vi "calculation vi_MD.vi"() -> ()   [LabVIEW 2012]
uses:
  Custom Controls/scan mode main settings tab.ctl
  Custom Controls/display palette control.ctl
  Custom Controls/pixel resolution enum.ctl
  Custom Controls/speed mode type def.ctl
  <vilib>/Utility/miscctls.llb/LVMinMaxIncTypeDef.ctl
  <vilib>/Utility/miscctls.llb/LVOutOfRangeActionTypeDef.ctl
  Custom Controls/experiment type.ctl
  Custom Controls/advanced settings inner tab CTL.ctl
  Custom Controls/MAIN Image panel tab Control type def.ctl
  Custom Controls/Histogram tab.ctl
  GFG/GFGnumericGet.vi
  GFG/GFGfpRefGet.vi
  GFG/GFGbooleanGet.vi
  GFG/GFGDisplayRefsGet.vi
  GFG/GFGImageRefsGet.vi
  GFG/GFG library.lvlib
panel:
  out "error out 3":errorcluster
  in  "String":string
  out "ready for flystart?":bool
  out "error out 2":errorcluster
  out "error out":errorcluster
  out "Source VI":string
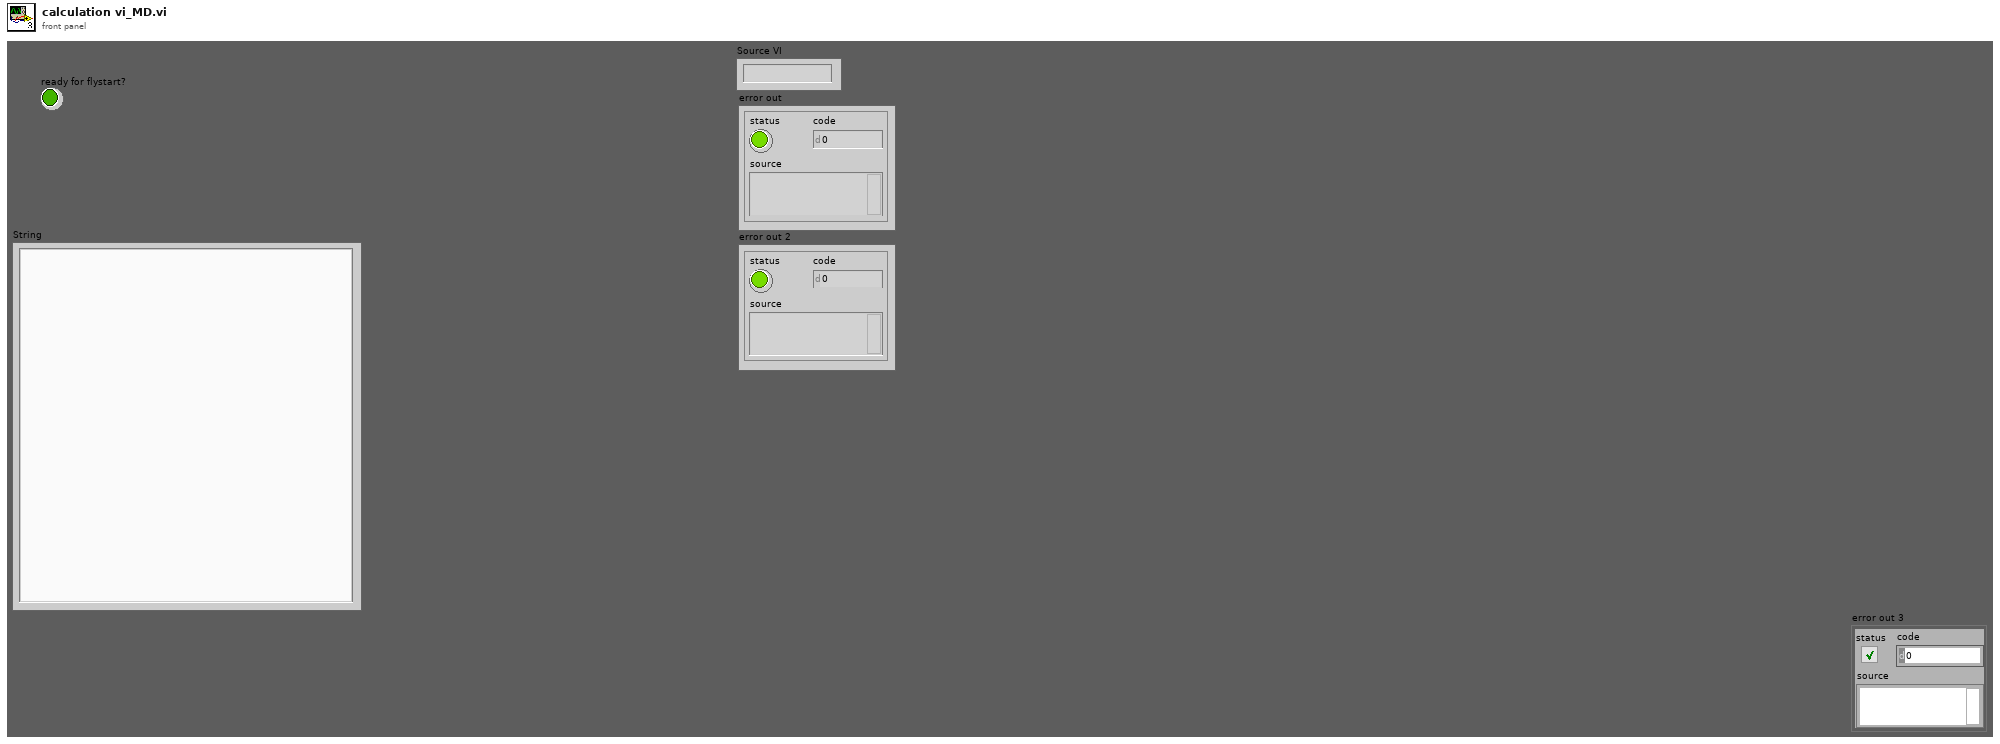
[diagram p1: front panel]
types:
  T1 = typedef "scan mode main settings tab.ctl" = enum32{"2D frame", "2D line scan", "general settings", "Z Stack", "piezo"}
  T2 = typedef "display palette control.ctl" = enum16{"standard", "high clipping red", "low clipping blue", "high and low clipping"}
  T3 = typedef "pixel resolution enum.ctl" = enum16{"   128 x 128", "   256 x 128", "   256 x 256", "   512 x  64", "   512 x 128", "   512 x 256", "   512 x 512", "  1024 x 512", "  1024 x 1024", "   arbitrary"}
  T4 = enum8{"Enabled", "Disabled", "Disabled and Grayed Out"}
  T5 = typedef "LVOutOfRangeActionTypeDef.ctl" = cluster{"Out of Range Action Minimum":u8, "Out of Range Action Maximum":u8, "Out of Range Action Increment":u8}
  T6 = typedef "LVMinMaxIncTypeDef.ctl" = cluster{"Minimum":dbl, "Maximum":dbl, "Increment":dbl}
  T7 = cluster{"xyvoltagefor2frames":dbl[][][], "x.pixels":dbl, "nomin.x.pixels":dbl, "y.pixels":dbl, "fill.fraction":dbl, "x.bidirectional":bool, "y.bidirectional":bool}
  T8 = typedef "experiment type.ctl" = string
  T9 = enum32{"Page Enabled", "Page Disabled", "Page Disabled & Grayed"}
  T10 = typedef "advanced settings inner tab CTL.ctl" = enum32{"arb. frames", "AO", "AI", "channels", "trigger", "Zstack data"}
  T11 = typedef "MAIN Image panel tab Control type def.ctl" = enum32{"Channel 1", "Channel 2", "Channel 3", "Channel 4", "all channels", "RGB overlay", "ROI", "arbitrary line scan"}
  T12 = typedef "Histogram tab.ctl" = enum32{"hist Ch 1", "hist Ch 4", "hist Ch 3", "hist Ch 2"}
  T13 = cluster{"WaveformChartRef":refnum<vi>, "DigitalRef":refnum<vi>, "ArrayRef":refnum<vi>, "TabControlRef":refnum<vi>, "EnumRef":refnum<vi>, "RingRef":refnum<vi>, "BooleanRef":refnum<vi>, "KnobRef":refnum<vi>, "SlideRef":refnum<vi>, "PathRef":refnum<vi>, "StringRef":refnum<vi>, "ComboBox":refnum<vi>, "WaveformGraphRef":refnum<vi>}
  T14 = cluster{"Channel 1 small":refnum<vi>, "Channel 2 small":refnum<vi>, "Channel 3 small":refnum<vi>, "Channel 4 small":refnum<vi>, "Channel 1 large":refnum<vi>, "Channel 2 large":refnum<vi>, "Channel 3 large":refnum<vi>, "Channel 4 large":refnum<vi>, "RGB overlay":refnum<vi>, "ROI Image display":refnum<vi>, "arb line scan display":refnum<vi>, "Channel 5 large":refnum<vi>}
  T15 = typedef "IMAQ Image.ctl" = refnum<image>
  T16 = cluster{"Channel 1 small":T15, "Channel 2 small":T15, "Channel 3 small":T15, "Channel 4 small":T15, "Channel 1 large":T15, "Channel 2 large":T15, "Channel 3 large":T15, "Channel 4 large":T15, "RGB overlay":T15, "ROI Image display":T15, "arb line scan display":T15, "Channel 5 large":T15}
  T17 = typedef "speed mode type def.ctl" = u16
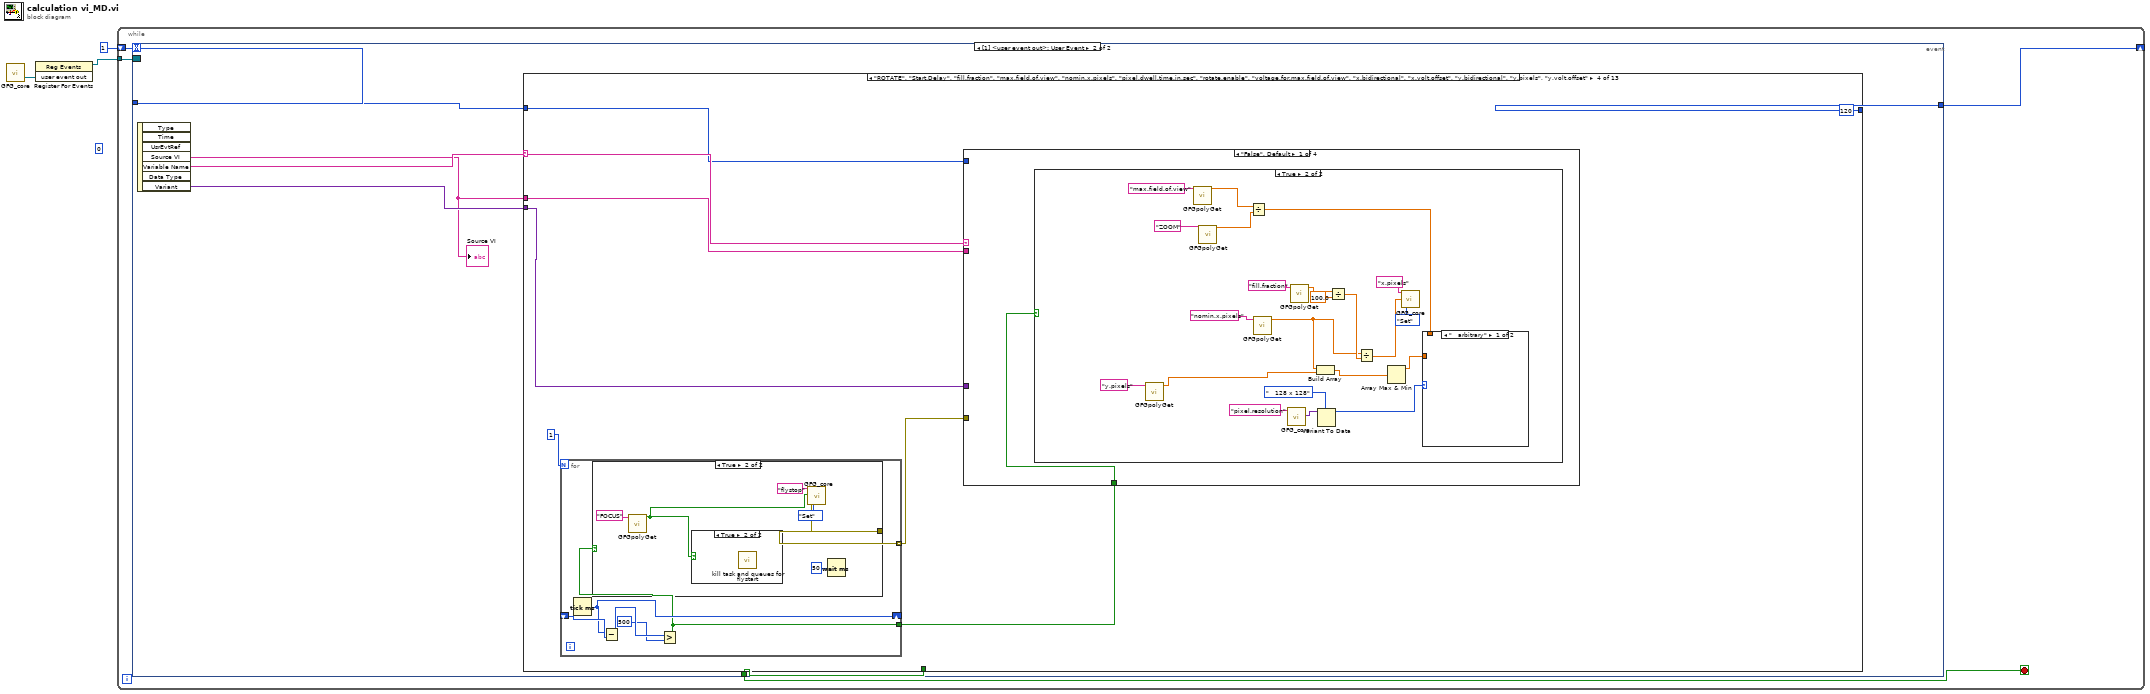
[diagram p0: block diagram]
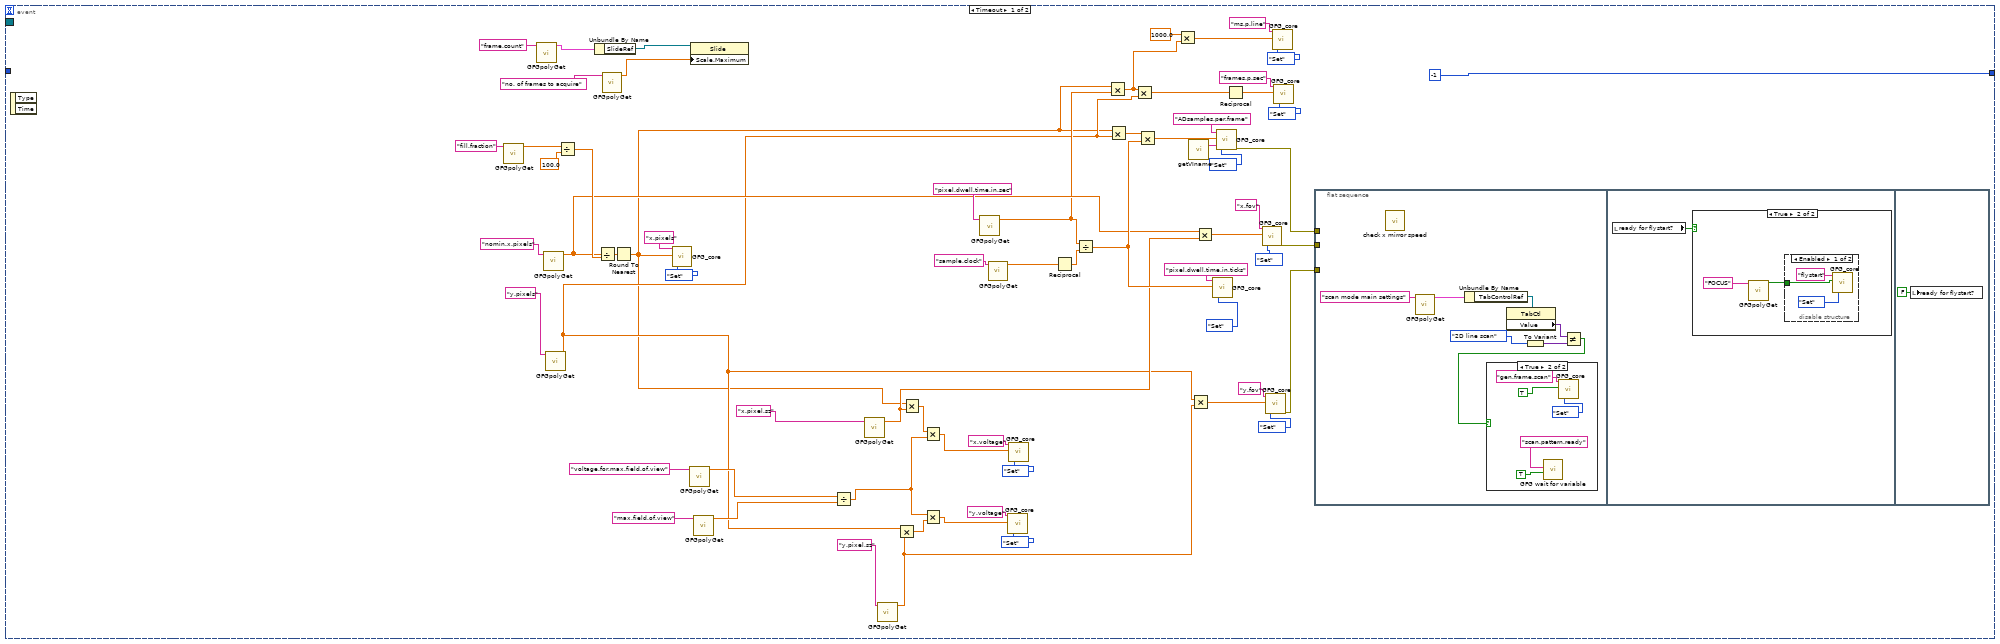
[diagram p2: hidden frame]
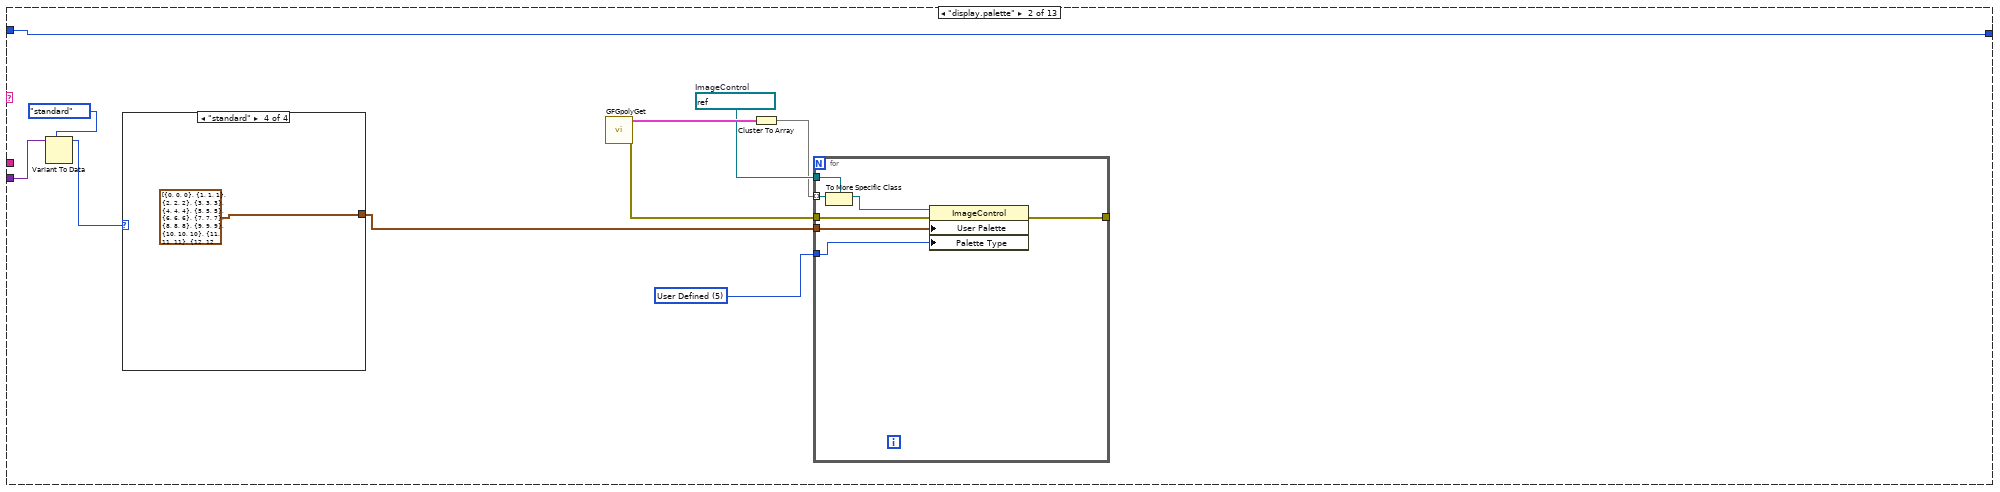
[diagram p7: hidden frame]
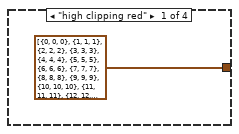
[diagram p8: hidden frame]
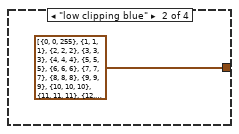
[diagram p9: hidden frame]
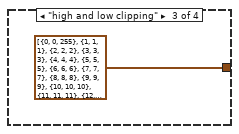
[diagram p10: hidden frame]
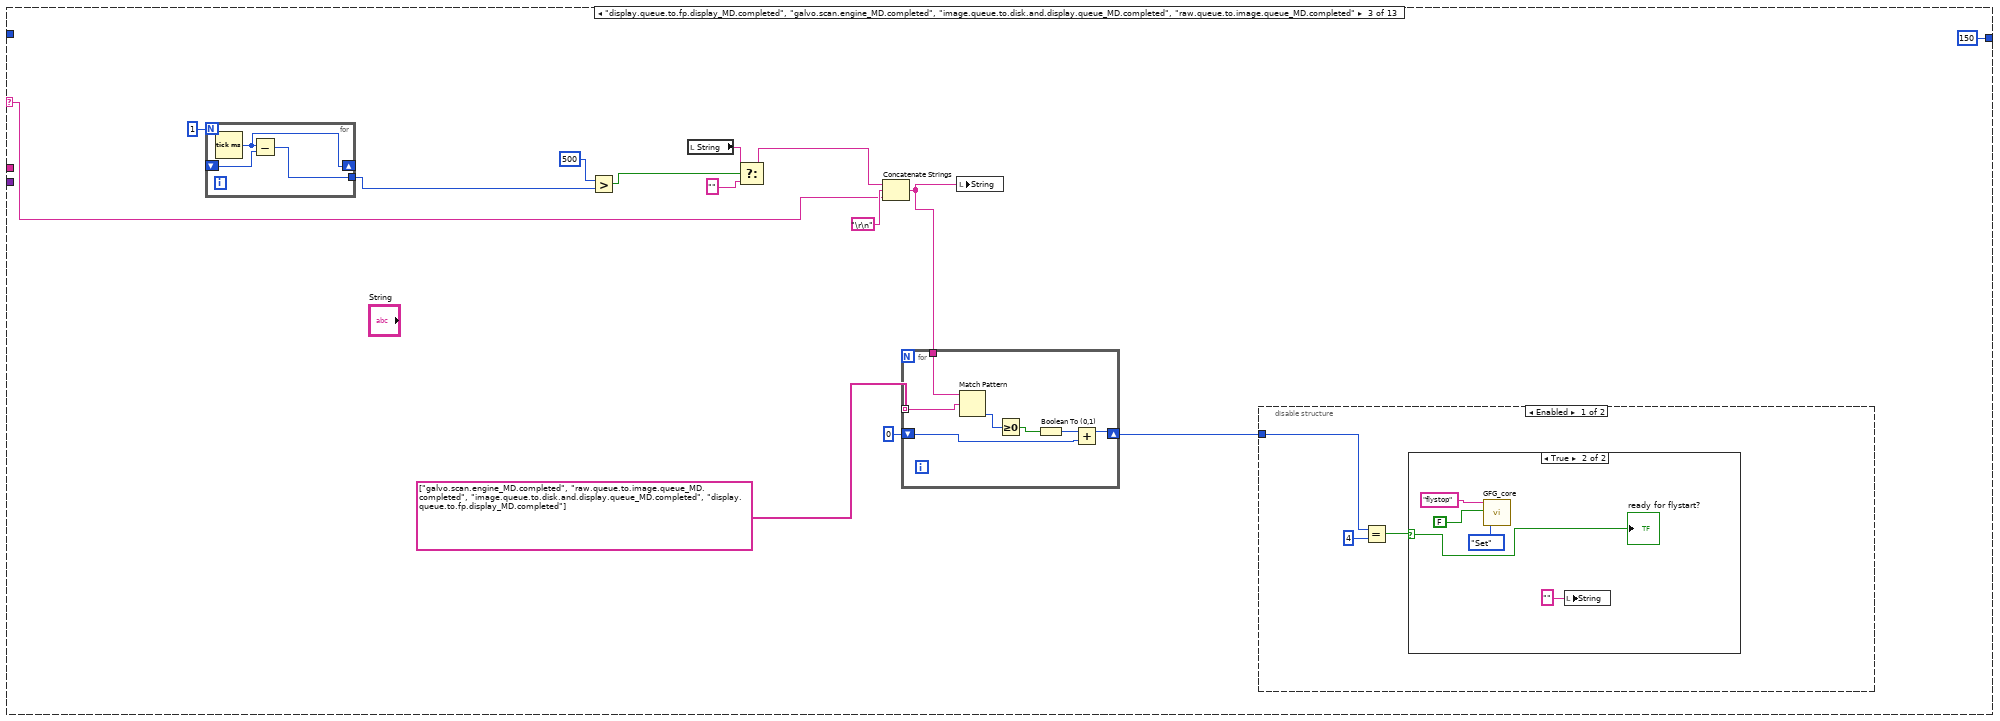
[diagram p11: hidden frame]
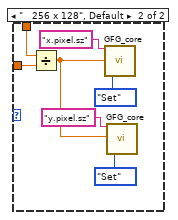
[diagram p17: hidden frame]
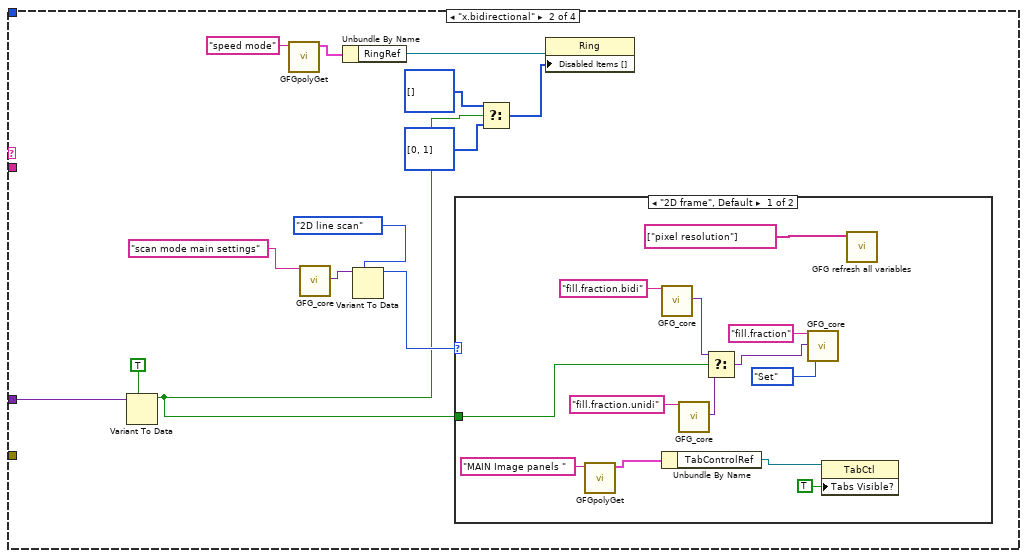
[diagram p18: hidden frame]
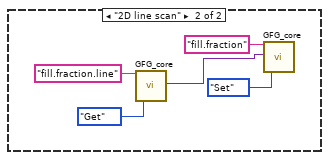
[diagram p19: hidden frame]
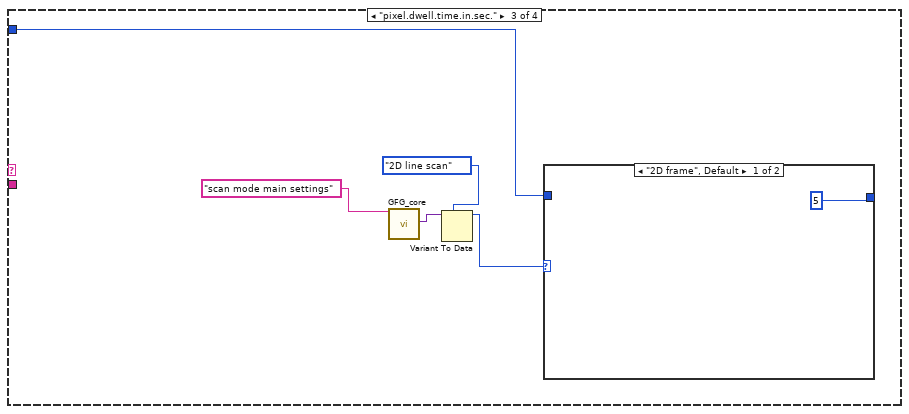
[diagram p20: hidden frame]
diagram:
  (unwired) 0
  n1 = call "GFG_core.vi"() -> ("user event out"=w3:refnum<user-event>)  [unwired: 13 in, 6 out]
  n2 = register-events(w3) -> (reference out=w2:refnum<event-registration>)  [unwired: 2 in, 1 out]
  n3 = while {
    tunnel: w2 -> [w7]
    shift-right: [w5] -> _
    shift-left: 1 -> [w4]
    stop <- w6 stop-if-true
    n4 = event shown="[1] <user event out>: User Event" {
      selector: w7 -> [_ _]
      dyn-events: _ -> [_ _]
      timeout: w4 -> [_ _]
      tunnel: [_ w97] -> w6
      tunnel: [-1 w95] -> w5
      tunnel: w4 -> [_ w94]
      event Timeout {
        n5 = event-data() -> ()  [unwired: 1 in, 2 out]
        n6 = call-poly "GFGpolyGet.vi"("Variable Name in"="fill.fraction") -> ("Numeric"=w53:dbl)  [unwired: 9 in, 1 out]
        n7 = call-poly "GFGpolyGet.vi"("Variable Name in"="frame.count") -> ("output cluster"=w14:T13)  [unwired: 9 in, 1 out]
        n8 = call-poly "GFGpolyGet.vi"("Variable Name in"="nomin.x.pixels") -> ("Numeric"=w29:dbl)  [unwired: 9 in, 1 out]
        n9 = call-poly "GFGpolyGet.vi"("Variable Name in"="y.pixels") -> ("Numeric"=w17:dbl)  [unwired: 9 in, 1 out]
        n10 = Divide(x=w53, y=100.0) -> (x/y=w49:dbl)
        n11 = Unbundle By Name(w14) -> ("SlideRef"=w13:refnum<vi>)
        n12 = Divide(x=w29, y=w49) -> (x/y=w30:dbl)
        n13 = call-poly "GFGpolyGet.vi"("Variable Name in"="no. of frames to acquire") -> ("Numeric"=w11:dbl)  [unwired: 9 in, 1 out]
        n14 = Round To Nearest(number=w30) -> (nearest integer value=w16:dbl)
        n15 = call "GFG_core.vi"("Variable Name in"="x.pixels", "Variant in"=w16, "Action"=enum16{"Init", "Set", "Get"}."Set") -> ()  [unwired: 10 in, 7 out]
        n16 = call-poly "GFGpolyGet.vi"("Variable Name in"="voltage.for.max.field.of.view") -> ("Numeric"=w44:dbl)  [unwired: 9 in, 1 out]
        n17 = property class="Slide"(reference=w13, "Scale.Maximum"=w11) -> ()  [unwired: 1 in, 2 out]
        n18 = call-poly "GFGpolyGet.vi"("Variable Name in"="max.field.of.view") -> ("Numeric"=w45:dbl)  [unwired: 9 in, 1 out]
        n19 = Divide(x=w44, y=w45) -> (x/y=w43:dbl)
        n20 = call-poly "GFGpolyGet.vi"("Variable Name in"="x.pixel.sz") -> ("Numeric"=w35:dbl)  [unwired: 9 in, 1 out]
        n21 = call-poly "GFGpolyGet.vi"("Variable Name in"="y.pixel.sz") -> ("Numeric"=w33:dbl)  [unwired: 9 in, 1 out]
        n22 = Multiply(x=w17, y=w33) -> (x*y=w32:dbl)
        n23 = Multiply(x=w16, y=w35) -> (x*y=w34:dbl)
        n24 = Multiply(x=w34, y=w43) -> (x*y=w38:dbl)
        n25 = Multiply(x=w43, y=w32) -> (x*y=w37:dbl)
        n26 = call-poly "GFGpolyGet.vi"("Variable Name in"="pixel.dwell.time.in.sec") -> ("Numeric"=w21:dbl)  [unwired: 9 in, 1 out]
        n27 = call-poly "GFGpolyGet.vi"("Variable Name in"="sample.clock") -> ("Numeric"=w31:dbl)  [unwired: 9 in, 1 out]
        n28 = call "GFG_core.vi"("Variable Name in"="y.voltage", "Variant in"=w37, "Action"=enum16{"Init", "Set", "Get"}."Set") -> ()  [unwired: 10 in, 7 out]
        n29 = call "GFG_core.vi"("Variable Name in"="x.voltage", "Variant in"=w38, "Action"=enum16{"Init", "Set", "Get"}."Set") -> ()  [unwired: 10 in, 7 out]
        n30 = Reciprocal(x=w31) -> (1/x=w60:dbl)
        n31 = Divide(x=w21, y=w60) -> (x/y=w56:dbl)
        n32 = Multiply(x=w16, y=w21) -> (x*y=w20:dbl)
        n33 = Multiply(x=w16, y=w17) -> (x*y=w28:dbl)
        n34 = Multiply(x=w20, y=w17) -> (x*y=w23:dbl)
        n35 = Multiply(x=w28, y=w56) -> (x*y=w72:dbl)
        n36 = Multiply(x=1000.0, y=w20) -> (x*y=w18:dbl)
        n37 = call "getVIname.vi"() -> ("VI name"=w70:string)  [unwired: 19 in]
        n38 = Multiply(x=w17, y=w33) -> (x*y=w62:dbl)
        n39 = Multiply(x=w29, y=w35) -> (x*y=w65:dbl)
        n40 = call "GFG_core.vi"("Variable Name in"="pixel.dwell.time.in.ticks", "Variant in"=w56, "Action"=enum16{"Init", "Set", "Get"}."Set") -> ()  [unwired: 10 in, 7 out]
        n41 = call "GFG_core.vi"("Variable Name in"="ADsamples.per.frame", "Variant in"=w72, "Source VI"=w70, "Action"=enum16{"Init", "Set", "Get"}."Set") -> ("error out"=w10:errorcluster)  [unwired: 9 in, 6 out]
        n42 = Reciprocal(x=w23) -> (1/x=w22:dbl)
        n43 = call "GFG_core.vi"("Variable Name in"="x.fov", "Variant in"=w65, "Action"=enum16{"Init", "Set", "Get"}."Set") -> ("error out"=w9:errorcluster)  [unwired: 10 in, 6 out]
        n44 = call "GFG_core.vi"("Variable Name in"="y.fov", "Variant in"=w62, "Action"=enum16{"Init", "Set", "Get"}."Set") -> ("error out"=w8:errorcluster)  [unwired: 10 in, 6 out]
        n45 = call "GFG_core.vi"("Variable Name in"="ms.p.line", "Variant in"=w18, "Action"=enum16{"Init", "Set", "Get"}."Set") -> ()  [unwired: 10 in, 7 out]
        n46 = call "GFG_core.vi"("Variable Name in"="frames.p.sec", "Variant in"=w22, "Action"=enum16{"Init", "Set", "Get"}."Set") -> ()  [unwired: 10 in, 7 out]
        n47 = flat-sequence {
          tunnel: w10 -> [_]
          tunnel: w9 -> [_]
          tunnel: w8 -> [_]
          frame #0 {
            n48 = call "check x mirror speed.vi"() -> ()  [unwired: 11 in, 1 out]
            n49 = call-poly "GFGpolyGet.vi"("Variable Name in"="scan mode main settings") -> ("output cluster"=w78:T13)  [unwired: 9 in, 1 out]
            n50 = Unbundle By Name(w78) -> ("TabControlRef"=w80:refnum<vi>)
            n51 = property class="TabCtl"(reference=w80) -> ("Value"=w77:variant)  [unwired: 1 in, 2 out]
            n52 = To Variant(anything=scan_mode_main_settings_tab."2D line scan" ("scan mode main settings")) -> (Variant=w75:variant)
            n53 = Not Equal?(x=w77, y=w75) -> (x != y?=w74:bool)
            n54 = case shown="True" w74 {
              frame False {
              }
              frame True {
                n55 = call "GFG wait for variable.vi"("Variant"=TRUE, "Variable Name"="scan.pattern.ready" ("Variable Name in")) -> ()  [unwired: 10 in]
                n56 = call "GFG_core.vi"("Variable Name in"="gen.frame.scan", "Variant in"=TRUE, "Action"=enum16{"Init", "Set", "Get"}."Set") -> ()  [unwired: 10 in, 7 out]
              }
            }
          }
          frame #1 {
            n57 = local read "ready for flystart?"() -> (w86:bool)
            n58 = case shown="True" w86 {
              frame False {
              }
              frame True {
                n59 = call-poly "GFGpolyGet.vi"("Variable Name in"="FOCUS") -> ("Boolean"=w87:bool)  [unwired: 10 in]
                n60 = disable-structure shown="Enabled" {
                  disable-tunnel: w87 -> [w89 _]
                  frame Enabled {
                    n61 = call "GFG_core.vi"("Variable Name in"="flystart", "Variant in"=w89, "Action"=enum16{"Init", "Set", "Get"}."Set") -> ()  [unwired: 10 in, 7 out]
                  }
                  frame Disabled {
                  }
                }
              }
            }
          }
          frame #2 {
            n62 = local write "ready for flystart?"(FALSE ("ready for flystart?")) -> ()
          }
        }
      }
      event User Event {
        n63 = event-data() -> ("Source VI"=w93:string, "Variable Name"=w98:string, "Variant"=w96:variant)  [unwired: 1 in, 4 out]
        "Source VI" <- w93
        n64 = case shown="\"ROTATE\", \"Start.Delay\", \"fill.fraction\", \"max.field.of.view\", \"nomin.x.pixels\", \"pixel.dwell.time.in.sec\", \"rotate.enable\", \"voltage.for.max.field.of.view\", \"x.bidirectional\", \"x.volt.offset\", \"y.bidirectional\", \"y.pixels\", \"y.volt.offset\"" w98 {
          selector: w98 -> [_ _ w122 w160 _ _ _ w285 _ _ _ _ _]
          tunnel: [_ _ _ _ _ _ _ _ _ _ _ _ TRUE] -> w97
          tunnel: w96 -> [_ w104 _ w159 _ w269 _ w287 _ w418 w478 w512 _]
          tunnel: [w99 w100 150 120 50 w267 w276 120 w404 w414 w475 w513 w514] -> w95
          tunnel: w94 -> [w99 w100 _ w158 _ w267 w276 _ w404 w415 w476 w513 w514]
          tunnel: w93 -> [_ _ _ w157 _ _ _ _ _ _ _ _ _]
          frame "False", Default {
          }
          frame "display.palette" {
            w105 = u32 5 items=["Grayscale", "Binary", "Gradient", "Rainbow", "Temperature", "User Defined"] ("Palette:Palette Type")
            w107 = refnum<vi> refnum  # ImageControl
            n65 = Variant To Data(type=display_palette_control."standard" ("display palette"), Variant=w104) -> (data=w102:T2)  [unwired: 1 in, 1 out]
            n66 = case shown="\"standard\"" w102 {
              tunnel: [cluster{"Red":u8, "Green":u8, "Blue":u8}[] [{"Red"=0, "Green"=0, "Blue"=0}, {"Red"=1, "Green"=1, "Blue"=1}, {"Red"=2, "Green"=2, "Blue"=2}, {"Red"=3, "Green"=3, "Blue"=3}, {"Red"=4, "Green"=4, "Blue"=4}, {"Red"=5, "Green"=5, "Blue"=5}, {"Red"=6, "Green"=6, "Blue"=6}, {"Red"=7, "Green"=7, "Blue"=7}, {"Red"=8, "Green"=8, "Blue"=8}, {"Red"=9, "Green"=9, "Blue"=9}, {"Red"=10, "Green"=10, "Blue"=10}, {"Red"=11, "Green"=11, "Blue"=11}, {"Red"=12, "Green"=12, "Blue"=12}, {"Red"=13, "Green"=13, "Blue"=13}, {"Red"=14, "Green"=14, "Blue"=14}, {"Red"=15, "Green"=15, "Blue"=15}, {"Red"=16, "Green"=16, "Blue"=16}, {"Red"=17, "Green"=17, "Blue"=17}, {"Red"=18, "Green"=18, "Blue"=18}, {"Red"=19, "Green"=19, "Blue"=19}, {"Red"=20, "Green"=20, "Blue"=20}, {"Red"=21, "Green"=21, "Blue"=21}, {"Red"=22, "Green"=22, "Blue"=22}, {"Red"=23, "Green"=23, "Blue"=23}, {"Red"=24, "Green"=24, "Blue"=24}, {"Red"=25, "Green"=25, "Blue"=25}, {"Red"=26, "Green"=26, "Blue"=26}, {"Red"=27, "Green"=27, "Blue"=27}, {"Red"=28, "Green"=28, "Blue"=28}, {"Red"=29, "Green"=29, "Blue"=29}, {"Red"=30, "Green"=30, "Blue"=30}, {"Red"=31, "Green"=31, "Blue"=31}, {"Red"=32, "Green"=32, "Blue"=32}, {"Red"=33, "Green"=33, "Blue"=33}, {"Red"=34, "Green"=34, "Blue"=34}, {"Red"=35, "Green"=35, "Blue"=35}, {"Red"=36, "Green"=36, "Blue"=36}, {"Red"=37, "Green"=37, "Blue"=37}, {"Red"=38, "Green"=38, "Blue"=38}, {"Red"=39, "Green"=39, "Blue"=39}, {"Red"=40, "Green"=40, "Blue"=40}, {"Red"=41, "Green"=41, "Blue"=41}, {"Red"=42, "Green"=42, "Blue"=42}, {"Red"=43, "Green"=43, "Blue"=43}, {"Red"=44, "Green"=44, "Blue"=44}, {"Red"=45, "Green"=45, "Blue"=45}, {"Red"=46, "Green"=46, "Blue"=46}, {"Red"=47, "Green"=47, "Blue"=47}, {"Red"=48, "Green"=48, "Blue"=48}, {"Red"=49, "Green"=49, "Blue"=49}, {"Red"=50, "Green"=50, "Blue"=50}, {"Red"=51, "Green"=51, "Blue"=51}, {"Red"=52, "Green"=52, "Blue"=52}, {"Red"=53, "Green"=53, "Blue"=53}, {"Red"=54, "Green"=54, "Blue"=54}, {"Red"=55, "Green"=55, "Blue"=55}, {"Red"=56, "Green"=56, "Blue"=56}, {"Red"=57, "Green"=57, "Blue"=57}, {"Red"=58, "Green"=58, "Blue"=58}, {"Red"=59, "Green"=59, "Blue"=59}, {"Red"=60, "Green"=60, "Blue"=60}, {"Red"=61, "Green"=61, "Blue"=61}, {"Red"=62, "Green"=62, "Blue"=62}, {"Red"=63, "Green"=63, "Blue"=63}, {"Red"=64, "Green"=64, "Blue"=64}, {"Red"=65, "Green"=65, "Blue"=65}, {"Red"=66, "Green"=66, "Blue"=66}, {"Red"=67, "Green"=67, "Blue"=67}, {"Red"=68, "Green"=68, "Blue"=68}, {"Red"=69, "Green"=69, "Blue"=69}, {"Red"=70, "Green"=70, "Blue"=70}, {"Red"=71, "Green"=71, "Blue"=71}, {"Red"=72, "Green"=72, "Blue"=72}, {"Red"=73, "Green"=73, "Blue"=73}, {"Red"=74, "Green"=74, "Blue"=74}, {"Red"=75, "Green"=75, "Blue"=75}, {"Red"=76, "Green"=76, "Blue"=76}, {"Red"=77, "Green"=77, "Blue"=77}, {"Red"=78, "Green"=78, "Blue"=78}, {"Red"=79, "Green"=79, "Blue"=79}, {"Red"=80, "Green"=80, "Blue"=80}, {"Red"=81, "Green"=81, "Blue"=81}, {"Red"=82, "Green"=82, "Blue"=82}, {"Red"=83, "Green"=83, "Blue"=83}, {"Red"=84, "Green"=84, "Blue"=84}, {"Red"=85, "Green"=85, "Blue"=85}, {"Red"=86, "Green"=86, "Blue"=86}, {"Red"=87, "Green"=87, "Blue"=87}, {"Red"=88, "Green"=88, "Blue"=88}, {"Red"=89, "Green"=89, "Blue"=89}, {"Red"=90, "Green"=90, "Blue"=90}, {"Red"=91, "Green"=91, "Blue"=91}, {"Red"=92, "Green"=92, "Blue"=92}, {"Red"=93, "Green"=93, "Blue"=93}, {"Red"=94, "Green"=94, "Blue"=94}, {"Red"=95, "Green"=95, "Blue"=95}, {"Red"=96, "Green"=96, "Blue"=96}, {"Red"=97, "Green"=97, "Blue"=97}, {"Red"=98, "Green"=98, "Blue"=98}, {"Red"=99, "Green"=99, "Blue"=99}, {"Red"=100, "Green"=100, "Blue"=100}, {"Red"=101, "Green"=101, "Blue"=101}, {"Red"=102, "Green"=102, "Blue"=102}, {"Red"=103, "Green"=103, "Blue"=103}, {"Red"=104, "Green"=104, "Blue"=104}, {"Red"=105, "Green"=105, "Blue"=105}, {"Red"=106, "Green"=106, "Blue"=106}, {"Red"=107, "Green"=107, "Blue"=107}, {"Red"=108, "Green"=108, "Blue"=108}, {"Red"=109, "Green"=109, "Blue"=109}, {"Red"=110, "Green"=110, "Blue"=110}, {"Red"=111, "Green"=111, "Blue"=111}, {"Red"=112, "Green"=112, "Blue"=112}, {"Red"=113, "Green"=113, "Blue"=113}, {"Red"=114, "Green"=114, "Blue"=114}, {"Red"=115, "Green"=115, "Blue"=115}, {"Red"=116, "Green"=116, "Blue"=116}, {"Red"=117, "Green"=117, "Blue"=117}, {"Red"=118, "Green"=118, "Blue"=118}, {"Red"=119, "Green"=119, "Blue"=119}, {"Red"=120, "Green"=120, "Blue"=120}, {"Red"=121, "Green"=121, "Blue"=121}, {"Red"=122, "Green"=122, "Blue"=122}, {"Red"=123, "Green"=123, "Blue"=123}, {"Red"=124, "Green"=124, "Blue"=124}, {"Red"=125, "Green"=125, "Blue"=125}, {"Red"=126, "Green"=126, "Blue"=126}, {"Red"=127, "Green"=127, "Blue"=127}, {"Red"=128, "Green"=128, "Blue"=128}, {"Red"=129, "Green"=129, "Blue"=129}, {"Red"=130, "Green"=130, "Blue"=130}, {"Red"=131, "Green"=131, "Blue"=131}, {"Red"=132, "Green"=132, "Blue"=132}, {"Red"=133, "Green"=133, "Blue"=133}, {"Red"=134, "Green"=134, "Blue"=134}, {"Red"=135, "Green"=135, "Blue"=135}, {"Red"=136, "Green"=136, "Blue"=136}, {"Red"=137, "Green"=137, "Blue"=137}, {"Red"=138, "Green"=138, "Blue"=138}, {"Red"=139, "Green"=139, "Blue"=139}, {"Red"=140, "Green"=140, "Blue"=140}, {"Red"=141, "Green"=141, "Blue"=141}, {"Red"=142, "Green"=142, "Blue"=142}, {"Red"=143, "Green"=143, "Blue"=143}, {"Red"=144, "Green"=144, "Blue"=144}, {"Red"=145, "Green"=145, "Blue"=145}, {"Red"=146, "Green"=146, "Blue"=146}, {"Red"=147, "Green"=147, "Blue"=147}, {"Red"=148, "Green"=148, "Blue"=148}, {"Red"=149, "Green"=149, "Blue"=149}, {"Red"=150, "Green"=150, "Blue"=150}, {"Red"=151, "Green"=151, "Blue"=151}, {"Red"=152, "Green"=152, "Blue"=152}, {"Red"=153, "Green"=153, "Blue"=153}, {"Red"=154, "Green"=154, "Blue"=154}, {"Red"=155, "Green"=155, "Blue"=155}, {"Red"=156, "Green"=156, "Blue"=156}, {"Red"=157, "Green"=157, "Blue"=157}, {"Red"=158, "Green"=158, "Blue"=158}, {"Red"=159, "Green"=159, "Blue"=159}, {"Red"=160, "Green"=160, "Blue"=160}, {"Red"=161, "Green"=161, "Blue"=161}, {"Red"=162, "Green"=162, "Blue"=162}, {"Red"=163, "Green"=163, "Blue"=163}, {"Red"=164, "Green"=164, "Blue"=164}, {"Red"=165, "Green"=165, "Blue"=165}, {"Red"=166, "Green"=166, "Blue"=166}, {"Red"=167, "Green"=167, "Blue"=167}, {"Red"=168, "Green"=168, "Blue"=168}, {"Red"=169, "Green"=169, "Blue"=169}, {"Red"=170, "Green"=170, "Blue"=170}, {"Red"=171, "Green"=171, "Blue"=171}, {"Red"=172, "Green"=172, "Blue"=172}, {"Red"=173, "Green"=173, "Blue"=173}, {"Red"=174, "Green"=174, "Blue"=174}, {"Red"=175, "Green"=175, "Blue"=175}, {"Red"=176, "Green"=176, "Blue"=176}, {"Red"=177, "Green"=177, "Blue"=177}, {"Red"=178, "Green"=178, "Blue"=178}, {"Red"=179, "Green"=179, "Blue"=179}, {"Red"=180, "Green"=180, "Blue"=180}, {"Red"=181, "Green"=181, "Blue"=181}, {"Red"=182, "Green"=182, "Blue"=182}, {"Red"=183, "Green"=183, "Blue"=183}, {"Red"=184, "Green"=184, "Blue"=184}, {"Red"=185, "Green"=185, "Blue"=185}, {"Red"=186, "Green"=186, "Blue"=186}, {"Red"=187, "Green"=187, "Blue"=187}, {"Red"=188, "Green"=188, "Blue"=188}, {"Red"=189, "Green"=189, "Blue"=189}, {"Red"=190, "Green"=190, "Blue"=190}, {"Red"=191, "Green"=191, "Blue"=191}, {"Red"=192, "Green"=192, "Blue"=192}, {"Red"=193, "Green"=193, "Blue"=193}, {"Red"=194, "Green"=194, "Blue"=194}, {"Red"=195, "Green"=195, "Blue"=195}, {"Red"=196, "Green"=196, "Blue"=196}, {"Red"=197, "Green"=197, "Blue"=197}, {"Red"=198, "Green"=198, "Blue"=198}, {"Red"=199, "Green"=199, "Blue"=199}, {"Red"=200, "Green"=200, "Blue"=200}, {"Red"=201, "Green"=201, "Blue"=201}, {"Red"=202, "Green"=202, "Blue"=202}, {"Red"=203, "Green"=203, "Blue"=203}, {"Red"=204, "Green"=204, "Blue"=204}, {"Red"=205, "Green"=205, "Blue"=205}, {"Red"=206, "Green"=206, "Blue"=206}, {"Red"=207, "Green"=207, "Blue"=207}, {"Red"=208, "Green"=208, "Blue"=208}, {"Red"=209, "Green"=209, "Blue"=209}, {"Red"=210, "Green"=210, "Blue"=210}, {"Red"=211, "Green"=211, "Blue"=211}, {"Red"=212, "Green"=212, "Blue"=212}, {"Red"=213, "Green"=213, "Blue"=213}, {"Red"=214, "Green"=214, "Blue"=214}, {"Red"=215, "Green"=215, "Blue"=215}, {"Red"=216, "Green"=216, "Blue"=216}, {"Red"=217, "Green"=217, "Blue"=217}, {"Red"=218, "Green"=218, "Blue"=218}, {"Red"=219, "Green"=219, "Blue"=219}, {"Red"=220, "Green"=220, "Blue"=220}, {"Red"=221, "Green"=221, "Blue"=221}, {"Red"=222, "Green"=222, "Blue"=222}, {"Red"=223, "Green"=223, "Blue"=223}, {"Red"=224, "Green"=224, "Blue"=224}, {"Red"=225, "Green"=225, "Blue"=225}, {"Red"=226, "Green"=226, "Blue"=226}, {"Red"=227, "Green"=227, "Blue"=227}, {"Red"=228, "Green"=228, "Blue"=228}, {"Red"=229, "Green"=229, "Blue"=229}, {"Red"=230, "Green"=230, "Blue"=230}, {"Red"=231, "Green"=231, "Blue"=231}, {"Red"=232, "Green"=232, "Blue"=232}, {"Red"=233, "Green"=233, "Blue"=233}, {"Red"=234, "Green"=234, "Blue"=234}, {"Red"=235, "Green"=235, "Blue"=235}, {"Red"=236, "Green"=236, "Blue"=236}, {"Red"=237, "Green"=237, "Blue"=237}, {"Red"=238, "Green"=238, "Blue"=238}, {"Red"=239, "Green"=239, "Blue"=239}, {"Red"=240, "Green"=240, "Blue"=240}, {"Red"=241, "Green"=241, "Blue"=241}, {"Red"=242, "Green"=242, "Blue"=242}, {"Red"=243, "Green"=243, "Blue"=243}, {"Red"=244, "Green"=244, "Blue"=244}, {"Red"=245, "Green"=245, "Blue"=245}, {"Red"=246, "Green"=246, "Blue"=246}, {"Red"=247, "Green"=247, "Blue"=247}, {"Red"=248, "Green"=248, "Blue"=248}, {"Red"=249, "Green"=249, "Blue"=249}, {"Red"=250, "Green"=250, "Blue"=250}, {"Red"=251, "Green"=251, "Blue"=251}, {"Red"=252, "Green"=252, "Blue"=252}, {"Red"=253, "Green"=253, "Blue"=253}, {"Red"=254, "Green"=254, "Blue"=254}, {"Red"=255, "Green"=0, "Blue"=0}] ("Color Palette") cluster{"Red":u8, "Green":u8, "Blue":u8}[] [{"Red"=0, "Green"=0, "Blue"=255}, {"Red"=1, "Green"=1, "Blue"=1}, {"Red"=2, "Green"=2, "Blue"=2}, {"Red"=3, "Green"=3, "Blue"=3}, {"Red"=4, "Green"=4, "Blue"=4}, {"Red"=5, "Green"=5, "Blue"=5}, {"Red"=6, "Green"=6, "Blue"=6}, {"Red"=7, "Green"=7, "Blue"=7}, {"Red"=8, "Green"=8, "Blue"=8}, {"Red"=9, "Green"=9, "Blue"=9}, {"Red"=10, "Green"=10, "Blue"=10}, {"Red"=11, "Green"=11, "Blue"=11}, {"Red"=12, "Green"=12, "Blue"=12}, {"Red"=13, "Green"=13, "Blue"=13}, {"Red"=14, "Green"=14, "Blue"=14}, {"Red"=15, "Green"=15, "Blue"=15}, {"Red"=16, "Green"=16, "Blue"=16}, {"Red"=17, "Green"=17, "Blue"=17}, {"Red"=18, "Green"=18, "Blue"=18}, {"Red"=19, "Green"=19, "Blue"=19}, {"Red"=20, "Green"=20, "Blue"=20}, {"Red"=21, "Green"=21, "Blue"=21}, {"Red"=22, "Green"=22, "Blue"=22}, {"Red"=23, "Green"=23, "Blue"=23}, {"Red"=24, "Green"=24, "Blue"=24}, {"Red"=25, "Green"=25, "Blue"=25}, {"Red"=26, "Green"=26, "Blue"=26}, {"Red"=27, "Green"=27, "Blue"=27}, {"Red"=28, "Green"=28, "Blue"=28}, {"Red"=29, "Green"=29, "Blue"=29}, {"Red"=30, "Green"=30, "Blue"=30}, {"Red"=31, "Green"=31, "Blue"=31}, {"Red"=32, "Green"=32, "Blue"=32}, {"Red"=33, "Green"=33, "Blue"=33}, {"Red"=34, "Green"=34, "Blue"=34}, {"Red"=35, "Green"=35, "Blue"=35}, {"Red"=36, "Green"=36, "Blue"=36}, {"Red"=37, "Green"=37, "Blue"=37}, {"Red"=38, "Green"=38, "Blue"=38}, {"Red"=39, "Green"=39, "Blue"=39}, {"Red"=40, "Green"=40, "Blue"=40}, {"Red"=41, "Green"=41, "Blue"=41}, {"Red"=42, "Green"=42, "Blue"=42}, {"Red"=43, "Green"=43, "Blue"=43}, {"Red"=44, "Green"=44, "Blue"=44}, {"Red"=45, "Green"=45, "Blue"=45}, {"Red"=46, "Green"=46, "Blue"=46}, {"Red"=47, "Green"=47, "Blue"=47}, {"Red"=48, "Green"=48, "Blue"=48}, {"Red"=49, "Green"=49, "Blue"=49}, {"Red"=50, "Green"=50, "Blue"=50}, {"Red"=51, "Green"=51, "Blue"=51}, {"Red"=52, "Green"=52, "Blue"=52}, {"Red"=53, "Green"=53, "Blue"=53}, {"Red"=54, "Green"=54, "Blue"=54}, {"Red"=55, "Green"=55, "Blue"=55}, {"Red"=56, "Green"=56, "Blue"=56}, {"Red"=57, "Green"=57, "Blue"=57}, {"Red"=58, "Green"=58, "Blue"=58}, {"Red"=59, "Green"=59, "Blue"=59}, {"Red"=60, "Green"=60, "Blue"=60}, {"Red"=61, "Green"=61, "Blue"=61}, {"Red"=62, "Green"=62, "Blue"=62}, {"Red"=63, "Green"=63, "Blue"=63}, {"Red"=64, "Green"=64, "Blue"=64}, {"Red"=65, "Green"=65, "Blue"=65}, {"Red"=66, "Green"=66, "Blue"=66}, {"Red"=67, "Green"=67, "Blue"=67}, {"Red"=68, "Green"=68, "Blue"=68}, {"Red"=69, "Green"=69, "Blue"=69}, {"Red"=70, "Green"=70, "Blue"=70}, {"Red"=71, "Green"=71, "Blue"=71}, {"Red"=72, "Green"=72, "Blue"=72}, {"Red"=73, "Green"=73, "Blue"=73}, {"Red"=74, "Green"=74, "Blue"=74}, {"Red"=75, "Green"=75, "Blue"=75}, {"Red"=76, "Green"=76, "Blue"=76}, {"Red"=77, "Green"=77, "Blue"=77}, {"Red"=78, "Green"=78, "Blue"=78}, {"Red"=79, "Green"=79, "Blue"=79}, {"Red"=80, "Green"=80, "Blue"=80}, {"Red"=81, "Green"=81, "Blue"=81}, {"Red"=82, "Green"=82, "Blue"=82}, {"Red"=83, "Green"=83, "Blue"=83}, {"Red"=84, "Green"=84, "Blue"=84}, {"Red"=85, "Green"=85, "Blue"=85}, {"Red"=86, "Green"=86, "Blue"=86}, {"Red"=87, "Green"=87, "Blue"=87}, {"Red"=88, "Green"=88, "Blue"=88}, {"Red"=89, "Green"=89, "Blue"=89}, {"Red"=90, "Green"=90, "Blue"=90}, {"Red"=91, "Green"=91, "Blue"=91}, {"Red"=92, "Green"=92, "Blue"=92}, {"Red"=93, "Green"=93, "Blue"=93}, {"Red"=94, "Green"=94, "Blue"=94}, {"Red"=95, "Green"=95, "Blue"=95}, {"Red"=96, "Green"=96, "Blue"=96}, {"Red"=97, "Green"=97, "Blue"=97}, {"Red"=98, "Green"=98, "Blue"=98}, {"Red"=99, "Green"=99, "Blue"=99}, {"Red"=100, "Green"=100, "Blue"=100}, {"Red"=101, "Green"=101, "Blue"=101}, {"Red"=102, "Green"=102, "Blue"=102}, {"Red"=103, "Green"=103, "Blue"=103}, {"Red"=104, "Green"=104, "Blue"=104}, {"Red"=105, "Green"=105, "Blue"=105}, {"Red"=106, "Green"=106, "Blue"=106}, {"Red"=107, "Green"=107, "Blue"=107}, {"Red"=108, "Green"=108, "Blue"=108}, {"Red"=109, "Green"=109, "Blue"=109}, {"Red"=110, "Green"=110, "Blue"=110}, {"Red"=111, "Green"=111, "Blue"=111}, {"Red"=112, "Green"=112, "Blue"=112}, {"Red"=113, "Green"=113, "Blue"=113}, {"Red"=114, "Green"=114, "Blue"=114}, {"Red"=115, "Green"=115, "Blue"=115}, {"Red"=116, "Green"=116, "Blue"=116}, {"Red"=117, "Green"=117, "Blue"=117}, {"Red"=118, "Green"=118, "Blue"=118}, {"Red"=119, "Green"=119, "Blue"=119}, {"Red"=120, "Green"=120, "Blue"=120}, {"Red"=121, "Green"=121, "Blue"=121}, {"Red"=122, "Green"=122, "Blue"=122}, {"Red"=123, "Green"=123, "Blue"=123}, {"Red"=124, "Green"=124, "Blue"=124}, {"Red"=125, "Green"=125, "Blue"=125}, {"Red"=126, "Green"=126, "Blue"=126}, {"Red"=127, "Green"=127, "Blue"=127}, {"Red"=128, "Green"=128, "Blue"=128}, {"Red"=129, "Green"=129, "Blue"=129}, {"Red"=130, "Green"=130, "Blue"=130}, {"Red"=131, "Green"=131, "Blue"=131}, {"Red"=132, "Green"=132, "Blue"=132}, {"Red"=133, "Green"=133, "Blue"=133}, {"Red"=134, "Green"=134, "Blue"=134}, {"Red"=135, "Green"=135, "Blue"=135}, {"Red"=136, "Green"=136, "Blue"=136}, {"Red"=137, "Green"=137, "Blue"=137}, {"Red"=138, "Green"=138, "Blue"=138}, {"Red"=139, "Green"=139, "Blue"=139}, {"Red"=140, "Green"=140, "Blue"=140}, {"Red"=141, "Green"=141, "Blue"=141}, {"Red"=142, "Green"=142, "Blue"=142}, {"Red"=143, "Green"=143, "Blue"=143}, {"Red"=144, "Green"=144, "Blue"=144}, {"Red"=145, "Green"=145, "Blue"=145}, {"Red"=146, "Green"=146, "Blue"=146}, {"Red"=147, "Green"=147, "Blue"=147}, {"Red"=148, "Green"=148, "Blue"=148}, {"Red"=149, "Green"=149, "Blue"=149}, {"Red"=150, "Green"=150, "Blue"=150}, {"Red"=151, "Green"=151, "Blue"=151}, {"Red"=152, "Green"=152, "Blue"=152}, {"Red"=153, "Green"=153, "Blue"=153}, {"Red"=154, "Green"=154, "Blue"=154}, {"Red"=155, "Green"=155, "Blue"=155}, {"Red"=156, "Green"=156, "Blue"=156}, {"Red"=157, "Green"=157, "Blue"=157}, {"Red"=158, "Green"=158, "Blue"=158}, {"Red"=159, "Green"=159, "Blue"=159}, {"Red"=160, "Green"=160, "Blue"=160}, {"Red"=161, "Green"=161, "Blue"=161}, {"Red"=162, "Green"=162, "Blue"=162}, {"Red"=163, "Green"=163, "Blue"=163}, {"Red"=164, "Green"=164, "Blue"=164}, {"Red"=165, "Green"=165, "Blue"=165}, {"Red"=166, "Green"=166, "Blue"=166}, {"Red"=167, "Green"=167, "Blue"=167}, {"Red"=168, "Green"=168, "Blue"=168}, {"Red"=169, "Green"=169, "Blue"=169}, {"Red"=170, "Green"=170, "Blue"=170}, {"Red"=171, "Green"=171, "Blue"=171}, {"Red"=172, "Green"=172, "Blue"=172}, {"Red"=173, "Green"=173, "Blue"=173}, {"Red"=174, "Green"=174, "Blue"=174}, {"Red"=175, "Green"=175, "Blue"=175}, {"Red"=176, "Green"=176, "Blue"=176}, {"Red"=177, "Green"=177, "Blue"=177}, {"Red"=178, "Green"=178, "Blue"=178}, {"Red"=179, "Green"=179, "Blue"=179}, {"Red"=180, "Green"=180, "Blue"=180}, {"Red"=181, "Green"=181, "Blue"=181}, {"Red"=182, "Green"=182, "Blue"=182}, {"Red"=183, "Green"=183, "Blue"=183}, {"Red"=184, "Green"=184, "Blue"=184}, {"Red"=185, "Green"=185, "Blue"=185}, {"Red"=186, "Green"=186, "Blue"=186}, {"Red"=187, "Green"=187, "Blue"=187}, {"Red"=188, "Green"=188, "Blue"=188}, {"Red"=189, "Green"=189, "Blue"=189}, {"Red"=190, "Green"=190, "Blue"=190}, {"Red"=191, "Green"=191, "Blue"=191}, {"Red"=192, "Green"=192, "Blue"=192}, {"Red"=193, "Green"=193, "Blue"=193}, {"Red"=194, "Green"=194, "Blue"=194}, {"Red"=195, "Green"=195, "Blue"=195}, {"Red"=196, "Green"=196, "Blue"=196}, {"Red"=197, "Green"=197, "Blue"=197}, {"Red"=198, "Green"=198, "Blue"=198}, {"Red"=199, "Green"=199, "Blue"=199}, {"Red"=200, "Green"=200, "Blue"=200}, {"Red"=201, "Green"=201, "Blue"=201}, {"Red"=202, "Green"=202, "Blue"=202}, {"Red"=203, "Green"=203, "Blue"=203}, {"Red"=204, "Green"=204, "Blue"=204}, {"Red"=205, "Green"=205, "Blue"=205}, {"Red"=206, "Green"=206, "Blue"=206}, {"Red"=207, "Green"=207, "Blue"=207}, {"Red"=208, "Green"=208, "Blue"=208}, {"Red"=209, "Green"=209, "Blue"=209}, {"Red"=210, "Green"=210, "Blue"=210}, {"Red"=211, "Green"=211, "Blue"=211}, {"Red"=212, "Green"=212, "Blue"=212}, {"Red"=213, "Green"=213, "Blue"=213}, {"Red"=214, "Green"=214, "Blue"=214}, {"Red"=215, "Green"=215, "Blue"=215}, {"Red"=216, "Green"=216, "Blue"=216}, {"Red"=217, "Green"=217, "Blue"=217}, {"Red"=218, "Green"=218, "Blue"=218}, {"Red"=219, "Green"=219, "Blue"=219}, {"Red"=220, "Green"=220, "Blue"=220}, {"Red"=221, "Green"=221, "Blue"=221}, {"Red"=222, "Green"=222, "Blue"=222}, {"Red"=223, "Green"=223, "Blue"=223}, {"Red"=224, "Green"=224, "Blue"=224}, {"Red"=225, "Green"=225, "Blue"=225}, {"Red"=226, "Green"=226, "Blue"=226}, {"Red"=227, "Green"=227, "Blue"=227}, {"Red"=228, "Green"=228, "Blue"=228}, {"Red"=229, "Green"=229, "Blue"=229}, {"Red"=230, "Green"=230, "Blue"=230}, {"Red"=231, "Green"=231, "Blue"=231}, {"Red"=232, "Green"=232, "Blue"=232}, {"Red"=233, "Green"=233, "Blue"=233}, {"Red"=234, "Green"=234, "Blue"=234}, {"Red"=235, "Green"=235, "Blue"=235}, {"Red"=236, "Green"=236, "Blue"=236}, {"Red"=237, "Green"=237, "Blue"=237}, {"Red"=238, "Green"=238, "Blue"=238}, {"Red"=239, "Green"=239, "Blue"=239}, {"Red"=240, "Green"=240, "Blue"=240}, {"Red"=241, "Green"=241, "Blue"=241}, {"Red"=242, "Green"=242, "Blue"=242}, {"Red"=243, "Green"=243, "Blue"=243}, {"Red"=244, "Green"=244, "Blue"=244}, {"Red"=245, "Green"=245, "Blue"=245}, {"Red"=246, "Green"=246, "Blue"=246}, {"Red"=247, "Green"=247, "Blue"=247}, {"Red"=248, "Green"=248, "Blue"=248}, {"Red"=249, "Green"=249, "Blue"=249}, {"Red"=250, "Green"=250, "Blue"=250}, {"Red"=251, "Green"=251, "Blue"=251}, {"Red"=252, "Green"=252, "Blue"=252}, {"Red"=253, "Green"=253, "Blue"=253}, {"Red"=254, "Green"=254, "Blue"=254}, {"Red"=255, "Green"=255, "Blue"=255}] ("Color Palette") cluster{"Red":u8, "Green":u8, "Blue":u8}[] [{"Red"=0, "Green"=0, "Blue"=255}, {"Red"=1, "Green"=1, "Blue"=1}, {"Red"=2, "Green"=2, "Blue"=2}, {"Red"=3, "Green"=3, "Blue"=3}, {"Red"=4, "Green"=4, "Blue"=4}, {"Red"=5, "Green"=5, "Blue"=5}, {"Red"=6, "Green"=6, "Blue"=6}, {"Red"=7, "Green"=7, "Blue"=7}, {"Red"=8, "Green"=8, "Blue"=8}, {"Red"=9, "Green"=9, "Blue"=9}, {"Red"=10, "Green"=10, "Blue"=10}, {"Red"=11, "Green"=11, "Blue"=11}, {"Red"=12, "Green"=12, "Blue"=12}, {"Red"=13, "Green"=13, "Blue"=13}, {"Red"=14, "Green"=14, "Blue"=14}, {"Red"=15, "Green"=15, "Blue"=15}, {"Red"=16, "Green"=16, "Blue"=16}, {"Red"=17, "Green"=17, "Blue"=17}, {"Red"=18, "Green"=18, "Blue"=18}, {"Red"=19, "Green"=19, "Blue"=19}, {"Red"=20, "Green"=20, "Blue"=20}, {"Red"=21, "Green"=21, "Blue"=21}, {"Red"=22, "Green"=22, "Blue"=22}, {"Red"=23, "Green"=23, "Blue"=23}, {"Red"=24, "Green"=24, "Blue"=24}, {"Red"=25, "Green"=25, "Blue"=25}, {"Red"=26, "Green"=26, "Blue"=26}, {"Red"=27, "Green"=27, "Blue"=27}, {"Red"=28, "Green"=28, "Blue"=28}, {"Red"=29, "Green"=29, "Blue"=29}, {"Red"=30, "Green"=30, "Blue"=30}, {"Red"=31, "Green"=31, "Blue"=31}, {"Red"=32, "Green"=32, "Blue"=32}, {"Red"=33, "Green"=33, "Blue"=33}, {"Red"=34, "Green"=34, "Blue"=34}, {"Red"=35, "Green"=35, "Blue"=35}, {"Red"=36, "Green"=36, "Blue"=36}, {"Red"=37, "Green"=37, "Blue"=37}, {"Red"=38, "Green"=38, "Blue"=38}, {"Red"=39, "Green"=39, "Blue"=39}, {"Red"=40, "Green"=40, "Blue"=40}, {"Red"=41, "Green"=41, "Blue"=41}, {"Red"=42, "Green"=42, "Blue"=42}, {"Red"=43, "Green"=43, "Blue"=43}, {"Red"=44, "Green"=44, "Blue"=44}, {"Red"=45, "Green"=45, "Blue"=45}, {"Red"=46, "Green"=46, "Blue"=46}, {"Red"=47, "Green"=47, "Blue"=47}, {"Red"=48, "Green"=48, "Blue"=48}, {"Red"=49, "Green"=49, "Blue"=49}, {"Red"=50, "Green"=50, "Blue"=50}, {"Red"=51, "Green"=51, "Blue"=51}, {"Red"=52, "Green"=52, "Blue"=52}, {"Red"=53, "Green"=53, "Blue"=53}, {"Red"=54, "Green"=54, "Blue"=54}, {"Red"=55, "Green"=55, "Blue"=55}, {"Red"=56, "Green"=56, "Blue"=56}, {"Red"=57, "Green"=57, "Blue"=57}, {"Red"=58, "Green"=58, "Blue"=58}, {"Red"=59, "Green"=59, "Blue"=59}, {"Red"=60, "Green"=60, "Blue"=60}, {"Red"=61, "Green"=61, "Blue"=61}, {"Red"=62, "Green"=62, "Blue"=62}, {"Red"=63, "Green"=63, "Blue"=63}, {"Red"=64, "Green"=64, "Blue"=64}, {"Red"=65, "Green"=65, "Blue"=65}, {"Red"=66, "Green"=66, "Blue"=66}, {"Red"=67, "Green"=67, "Blue"=67}, {"Red"=68, "Green"=68, "Blue"=68}, {"Red"=69, "Green"=69, "Blue"=69}, {"Red"=70, "Green"=70, "Blue"=70}, {"Red"=71, "Green"=71, "Blue"=71}, {"Red"=72, "Green"=72, "Blue"=72}, {"Red"=73, "Green"=73, "Blue"=73}, {"Red"=74, "Green"=74, "Blue"=74}, {"Red"=75, "Green"=75, "Blue"=75}, {"Red"=76, "Green"=76, "Blue"=76}, {"Red"=77, "Green"=77, "Blue"=77}, {"Red"=78, "Green"=78, "Blue"=78}, {"Red"=79, "Green"=79, "Blue"=79}, {"Red"=80, "Green"=80, "Blue"=80}, {"Red"=81, "Green"=81, "Blue"=81}, {"Red"=82, "Green"=82, "Blue"=82}, {"Red"=83, "Green"=83, "Blue"=83}, {"Red"=84, "Green"=84, "Blue"=84}, {"Red"=85, "Green"=85, "Blue"=85}, {"Red"=86, "Green"=86, "Blue"=86}, {"Red"=87, "Green"=87, "Blue"=87}, {"Red"=88, "Green"=88, "Blue"=88}, {"Red"=89, "Green"=89, "Blue"=89}, {"Red"=90, "Green"=90, "Blue"=90}, {"Red"=91, "Green"=91, "Blue"=91}, {"Red"=92, "Green"=92, "Blue"=92}, {"Red"=93, "Green"=93, "Blue"=93}, {"Red"=94, "Green"=94, "Blue"=94}, {"Red"=95, "Green"=95, "Blue"=95}, {"Red"=96, "Green"=96, "Blue"=96}, {"Red"=97, "Green"=97, "Blue"=97}, {"Red"=98, "Green"=98, "Blue"=98}, {"Red"=99, "Green"=99, "Blue"=99}, {"Red"=100, "Green"=100, "Blue"=100}, {"Red"=101, "Green"=101, "Blue"=101}, {"Red"=102, "Green"=102, "Blue"=102}, {"Red"=103, "Green"=103, "Blue"=103}, {"Red"=104, "Green"=104, "Blue"=104}, {"Red"=105, "Green"=105, "Blue"=105}, {"Red"=106, "Green"=106, "Blue"=106}, {"Red"=107, "Green"=107, "Blue"=107}, {"Red"=108, "Green"=108, "Blue"=108}, {"Red"=109, "Green"=109, "Blue"=109}, {"Red"=110, "Green"=110, "Blue"=110}, {"Red"=111, "Green"=111, "Blue"=111}, {"Red"=112, "Green"=112, "Blue"=112}, {"Red"=113, "Green"=113, "Blue"=113}, {"Red"=114, "Green"=114, "Blue"=114}, {"Red"=115, "Green"=115, "Blue"=115}, {"Red"=116, "Green"=116, "Blue"=116}, {"Red"=117, "Green"=117, "Blue"=117}, {"Red"=118, "Green"=118, "Blue"=118}, {"Red"=119, "Green"=119, "Blue"=119}, {"Red"=120, "Green"=120, "Blue"=120}, {"Red"=121, "Green"=121, "Blue"=121}, {"Red"=122, "Green"=122, "Blue"=122}, {"Red"=123, "Green"=123, "Blue"=123}, {"Red"=124, "Green"=124, "Blue"=124}, {"Red"=125, "Green"=125, "Blue"=125}, {"Red"=126, "Green"=126, "Blue"=126}, {"Red"=127, "Green"=127, "Blue"=127}, {"Red"=128, "Green"=128, "Blue"=128}, {"Red"=129, "Green"=129, "Blue"=129}, {"Red"=130, "Green"=130, "Blue"=130}, {"Red"=131, "Green"=131, "Blue"=131}, {"Red"=132, "Green"=132, "Blue"=132}, {"Red"=133, "Green"=133, "Blue"=133}, {"Red"=134, "Green"=134, "Blue"=134}, {"Red"=135, "Green"=135, "Blue"=135}, {"Red"=136, "Green"=136, "Blue"=136}, {"Red"=137, "Green"=137, "Blue"=137}, {"Red"=138, "Green"=138, "Blue"=138}, {"Red"=139, "Green"=139, "Blue"=139}, {"Red"=140, "Green"=140, "Blue"=140}, {"Red"=141, "Green"=141, "Blue"=141}, {"Red"=142, "Green"=142, "Blue"=142}, {"Red"=143, "Green"=143, "Blue"=143}, {"Red"=144, "Green"=144, "Blue"=144}, {"Red"=145, "Green"=145, "Blue"=145}, {"Red"=146, "Green"=146, "Blue"=146}, {"Red"=147, "Green"=147, "Blue"=147}, {"Red"=148, "Green"=148, "Blue"=148}, {"Red"=149, "Green"=149, "Blue"=149}, {"Red"=150, "Green"=150, "Blue"=150}, {"Red"=151, "Green"=151, "Blue"=151}, {"Red"=152, "Green"=152, "Blue"=152}, {"Red"=153, "Green"=153, "Blue"=153}, {"Red"=154, "Green"=154, "Blue"=154}, {"Red"=155, "Green"=155, "Blue"=155}, {"Red"=156, "Green"=156, "Blue"=156}, {"Red"=157, "Green"=157, "Blue"=157}, {"Red"=158, "Green"=158, "Blue"=158}, {"Red"=159, "Green"=159, "Blue"=159}, {"Red"=160, "Green"=160, "Blue"=160}, {"Red"=161, "Green"=161, "Blue"=161}, {"Red"=162, "Green"=162, "Blue"=162}, {"Red"=163, "Green"=163, "Blue"=163}, {"Red"=164, "Green"=164, "Blue"=164}, {"Red"=165, "Green"=165, "Blue"=165}, {"Red"=166, "Green"=166, "Blue"=166}, {"Red"=167, "Green"=167, "Blue"=167}, {"Red"=168, "Green"=168, "Blue"=168}, {"Red"=169, "Green"=169, "Blue"=169}, {"Red"=170, "Green"=170, "Blue"=170}, {"Red"=171, "Green"=171, "Blue"=171}, {"Red"=172, "Green"=172, "Blue"=172}, {"Red"=173, "Green"=173, "Blue"=173}, {"Red"=174, "Green"=174, "Blue"=174}, {"Red"=175, "Green"=175, "Blue"=175}, {"Red"=176, "Green"=176, "Blue"=176}, {"Red"=177, "Green"=177, "Blue"=177}, {"Red"=178, "Green"=178, "Blue"=178}, {"Red"=179, "Green"=179, "Blue"=179}, {"Red"=180, "Green"=180, "Blue"=180}, {"Red"=181, "Green"=181, "Blue"=181}, {"Red"=182, "Green"=182, "Blue"=182}, {"Red"=183, "Green"=183, "Blue"=183}, {"Red"=184, "Green"=184, "Blue"=184}, {"Red"=185, "Green"=185, "Blue"=185}, {"Red"=186, "Green"=186, "Blue"=186}, {"Red"=187, "Green"=187, "Blue"=187}, {"Red"=188, "Green"=188, "Blue"=188}, {"Red"=189, "Green"=189, "Blue"=189}, {"Red"=190, "Green"=190, "Blue"=190}, {"Red"=191, "Green"=191, "Blue"=191}, {"Red"=192, "Green"=192, "Blue"=192}, {"Red"=193, "Green"=193, "Blue"=193}, {"Red"=194, "Green"=194, "Blue"=194}, {"Red"=195, "Green"=195, "Blue"=195}, {"Red"=196, "Green"=196, "Blue"=196}, {"Red"=197, "Green"=197, "Blue"=197}, {"Red"=198, "Green"=198, "Blue"=198}, {"Red"=199, "Green"=199, "Blue"=199}, {"Red"=200, "Green"=200, "Blue"=200}, {"Red"=201, "Green"=201, "Blue"=201}, {"Red"=202, "Green"=202, "Blue"=202}, {"Red"=203, "Green"=203, "Blue"=203}, {"Red"=204, "Green"=204, "Blue"=204}, {"Red"=205, "Green"=205, "Blue"=205}, {"Red"=206, "Green"=206, "Blue"=206}, {"Red"=207, "Green"=207, "Blue"=207}, {"Red"=208, "Green"=208, "Blue"=208}, {"Red"=209, "Green"=209, "Blue"=209}, {"Red"=210, "Green"=210, "Blue"=210}, {"Red"=211, "Green"=211, "Blue"=211}, {"Red"=212, "Green"=212, "Blue"=212}, {"Red"=213, "Green"=213, "Blue"=213}, {"Red"=214, "Green"=214, "Blue"=214}, {"Red"=215, "Green"=215, "Blue"=215}, {"Red"=216, "Green"=216, "Blue"=216}, {"Red"=217, "Green"=217, "Blue"=217}, {"Red"=218, "Green"=218, "Blue"=218}, {"Red"=219, "Green"=219, "Blue"=219}, {"Red"=220, "Green"=220, "Blue"=220}, {"Red"=221, "Green"=221, "Blue"=221}, {"Red"=222, "Green"=222, "Blue"=222}, {"Red"=223, "Green"=223, "Blue"=223}, {"Red"=224, "Green"=224, "Blue"=224}, {"Red"=225, "Green"=225, "Blue"=225}, {"Red"=226, "Green"=226, "Blue"=226}, {"Red"=227, "Green"=227, "Blue"=227}, {"Red"=228, "Green"=228, "Blue"=228}, {"Red"=229, "Green"=229, "Blue"=229}, {"Red"=230, "Green"=230, "Blue"=230}, {"Red"=231, "Green"=231, "Blue"=231}, {"Red"=232, "Green"=232, "Blue"=232}, {"Red"=233, "Green"=233, "Blue"=233}, {"Red"=234, "Green"=234, "Blue"=234}, {"Red"=235, "Green"=235, "Blue"=235}, {"Red"=236, "Green"=236, "Blue"=236}, {"Red"=237, "Green"=237, "Blue"=237}, {"Red"=238, "Green"=238, "Blue"=238}, {"Red"=239, "Green"=239, "Blue"=239}, {"Red"=240, "Green"=240, "Blue"=240}, {"Red"=241, "Green"=241, "Blue"=241}, {"Red"=242, "Green"=242, "Blue"=242}, {"Red"=243, "Green"=243, "Blue"=243}, {"Red"=244, "Green"=244, "Blue"=244}, {"Red"=245, "Green"=245, "Blue"=245}, {"Red"=246, "Green"=246, "Blue"=246}, {"Red"=247, "Green"=247, "Blue"=247}, {"Red"=248, "Green"=248, "Blue"=248}, {"Red"=249, "Green"=249, "Blue"=249}, {"Red"=250, "Green"=250, "Blue"=250}, {"Red"=251, "Green"=251, "Blue"=251}, {"Red"=252, "Green"=252, "Blue"=252}, {"Red"=253, "Green"=253, "Blue"=253}, {"Red"=254, "Green"=254, "Blue"=254}, {"Red"=255, "Green"=0, "Blue"=0}] ("Color Palette") cluster{"Red":u8, "Green":u8, "Blue":u8}[] [{"Red"=0, "Green"=0, "Blue"=0}, {"Red"=1, "Green"=1, "Blue"=1}, {"Red"=2, "Green"=2, "Blue"=2}, {"Red"=3, "Green"=3, "Blue"=3}, {"Red"=4, "Green"=4, "Blue"=4}, {"Red"=5, "Green"=5, "Blue"=5}, {"Red"=6, "Green"=6, "Blue"=6}, {"Red"=7, "Green"=7, "Blue"=7}, {"Red"=8, "Green"=8, "Blue"=8}, {"Red"=9, "Green"=9, "Blue"=9}, {"Red"=10, "Green"=10, "Blue"=10}, {"Red"=11, "Green"=11, "Blue"=11}, {"Red"=12, "Green"=12, "Blue"=12}, {"Red"=13, "Green"=13, "Blue"=13}, {"Red"=14, "Green"=14, "Blue"=14}, {"Red"=15, "Green"=15, "Blue"=15}, {"Red"=16, "Green"=16, "Blue"=16}, {"Red"=17, "Green"=17, "Blue"=17}, {"Red"=18, "Green"=18, "Blue"=18}, {"Red"=19, "Green"=19, "Blue"=19}, {"Red"=20, "Green"=20, "Blue"=20}, {"Red"=21, "Green"=21, "Blue"=21}, {"Red"=22, "Green"=22, "Blue"=22}, {"Red"=23, "Green"=23, "Blue"=23}, {"Red"=24, "Green"=24, "Blue"=24}, {"Red"=25, "Green"=25, "Blue"=25}, {"Red"=26, "Green"=26, "Blue"=26}, {"Red"=27, "Green"=27, "Blue"=27}, {"Red"=28, "Green"=28, "Blue"=28}, {"Red"=29, "Green"=29, "Blue"=29}, {"Red"=30, "Green"=30, "Blue"=30}, {"Red"=31, "Green"=31, "Blue"=31}, {"Red"=32, "Green"=32, "Blue"=32}, {"Red"=33, "Green"=33, "Blue"=33}, {"Red"=34, "Green"=34, "Blue"=34}, {"Red"=35, "Green"=35, "Blue"=35}, {"Red"=36, "Green"=36, "Blue"=36}, {"Red"=37, "Green"=37, "Blue"=37}, {"Red"=38, "Green"=38, "Blue"=38}, {"Red"=39, "Green"=39, "Blue"=39}, {"Red"=40, "Green"=40, "Blue"=40}, {"Red"=41, "Green"=41, "Blue"=41}, {"Red"=42, "Green"=42, "Blue"=42}, {"Red"=43, "Green"=43, "Blue"=43}, {"Red"=44, "Green"=44, "Blue"=44}, {"Red"=45, "Green"=45, "Blue"=45}, {"Red"=46, "Green"=46, "Blue"=46}, {"Red"=47, "Green"=47, "Blue"=47}, {"Red"=48, "Green"=48, "Blue"=48}, {"Red"=49, "Green"=49, "Blue"=49}, {"Red"=50, "Green"=50, "Blue"=50}, {"Red"=51, "Green"=51, "Blue"=51}, {"Red"=52, "Green"=52, "Blue"=52}, {"Red"=53, "Green"=53, "Blue"=53}, {"Red"=54, "Green"=54, "Blue"=54}, {"Red"=55, "Green"=55, "Blue"=55}, {"Red"=56, "Green"=56, "Blue"=56}, {"Red"=57, "Green"=57, "Blue"=57}, {"Red"=58, "Green"=58, "Blue"=58}, {"Red"=59, "Green"=59, "Blue"=59}, {"Red"=60, "Green"=60, "Blue"=60}, {"Red"=61, "Green"=61, "Blue"=61}, {"Red"=62, "Green"=62, "Blue"=62}, {"Red"=63, "Green"=63, "Blue"=63}, {"Red"=64, "Green"=64, "Blue"=64}, {"Red"=65, "Green"=65, "Blue"=65}, {"Red"=66, "Green"=66, "Blue"=66}, {"Red"=67, "Green"=67, "Blue"=67}, {"Red"=68, "Green"=68, "Blue"=68}, {"Red"=69, "Green"=69, "Blue"=69}, {"Red"=70, "Green"=70, "Blue"=70}, {"Red"=71, "Green"=71, "Blue"=71}, {"Red"=72, "Green"=72, "Blue"=72}, {"Red"=73, "Green"=73, "Blue"=73}, {"Red"=74, "Green"=74, "Blue"=74}, {"Red"=75, "Green"=75, "Blue"=75}, {"Red"=76, "Green"=76, "Blue"=76}, {"Red"=77, "Green"=77, "Blue"=77}, {"Red"=78, "Green"=78, "Blue"=78}, {"Red"=79, "Green"=79, "Blue"=79}, {"Red"=80, "Green"=80, "Blue"=80}, {"Red"=81, "Green"=81, "Blue"=81}, {"Red"=82, "Green"=82, "Blue"=82}, {"Red"=83, "Green"=83, "Blue"=83}, {"Red"=84, "Green"=84, "Blue"=84}, {"Red"=85, "Green"=85, "Blue"=85}, {"Red"=86, "Green"=86, "Blue"=86}, {"Red"=87, "Green"=87, "Blue"=87}, {"Red"=88, "Green"=88, "Blue"=88}, {"Red"=89, "Green"=89, "Blue"=89}, {"Red"=90, "Green"=90, "Blue"=90}, {"Red"=91, "Green"=91, "Blue"=91}, {"Red"=92, "Green"=92, "Blue"=92}, {"Red"=93, "Green"=93, "Blue"=93}, {"Red"=94, "Green"=94, "Blue"=94}, {"Red"=95, "Green"=95, "Blue"=95}, {"Red"=96, "Green"=96, "Blue"=96}, {"Red"=97, "Green"=97, "Blue"=97}, {"Red"=98, "Green"=98, "Blue"=98}, {"Red"=99, "Green"=99, "Blue"=99}, {"Red"=100, "Green"=100, "Blue"=100}, {"Red"=101, "Green"=101, "Blue"=101}, {"Red"=102, "Green"=102, "Blue"=102}, {"Red"=103, "Green"=103, "Blue"=103}, {"Red"=104, "Green"=104, "Blue"=104}, {"Red"=105, "Green"=105, "Blue"=105}, {"Red"=106, "Green"=106, "Blue"=106}, {"Red"=107, "Green"=107, "Blue"=107}, {"Red"=108, "Green"=108, "Blue"=108}, {"Red"=109, "Green"=109, "Blue"=109}, {"Red"=110, "Green"=110, "Blue"=110}, {"Red"=111, "Green"=111, "Blue"=111}, {"Red"=112, "Green"=112, "Blue"=112}, {"Red"=113, "Green"=113, "Blue"=113}, {"Red"=114, "Green"=114, "Blue"=114}, {"Red"=115, "Green"=115, "Blue"=115}, {"Red"=116, "Green"=116, "Blue"=116}, {"Red"=117, "Green"=117, "Blue"=117}, {"Red"=118, "Green"=118, "Blue"=118}, {"Red"=119, "Green"=119, "Blue"=119}, {"Red"=120, "Green"=120, "Blue"=120}, {"Red"=121, "Green"=121, "Blue"=121}, {"Red"=122, "Green"=122, "Blue"=122}, {"Red"=123, "Green"=123, "Blue"=123}, {"Red"=124, "Green"=124, "Blue"=124}, {"Red"=125, "Green"=125, "Blue"=125}, {"Red"=126, "Green"=126, "Blue"=126}, {"Red"=127, "Green"=127, "Blue"=127}, {"Red"=128, "Green"=128, "Blue"=128}, {"Red"=129, "Green"=129, "Blue"=129}, {"Red"=130, "Green"=130, "Blue"=130}, {"Red"=131, "Green"=131, "Blue"=131}, {"Red"=132, "Green"=132, "Blue"=132}, {"Red"=133, "Green"=133, "Blue"=133}, {"Red"=134, "Green"=134, "Blue"=134}, {"Red"=135, "Green"=135, "Blue"=135}, {"Red"=136, "Green"=136, "Blue"=136}, {"Red"=137, "Green"=137, "Blue"=137}, {"Red"=138, "Green"=138, "Blue"=138}, {"Red"=139, "Green"=139, "Blue"=139}, {"Red"=140, "Green"=140, "Blue"=140}, {"Red"=141, "Green"=141, "Blue"=141}, {"Red"=142, "Green"=142, "Blue"=142}, {"Red"=143, "Green"=143, "Blue"=143}, {"Red"=144, "Green"=144, "Blue"=144}, {"Red"=145, "Green"=145, "Blue"=145}, {"Red"=146, "Green"=146, "Blue"=146}, {"Red"=147, "Green"=147, "Blue"=147}, {"Red"=148, "Green"=148, "Blue"=148}, {"Red"=149, "Green"=149, "Blue"=149}, {"Red"=150, "Green"=150, "Blue"=150}, {"Red"=151, "Green"=151, "Blue"=151}, {"Red"=152, "Green"=152, "Blue"=152}, {"Red"=153, "Green"=153, "Blue"=153}, {"Red"=154, "Green"=154, "Blue"=154}, {"Red"=155, "Green"=155, "Blue"=155}, {"Red"=156, "Green"=156, "Blue"=156}, {"Red"=157, "Green"=157, "Blue"=157}, {"Red"=158, "Green"=158, "Blue"=158}, {"Red"=159, "Green"=159, "Blue"=159}, {"Red"=160, "Green"=160, "Blue"=160}, {"Red"=161, "Green"=161, "Blue"=161}, {"Red"=162, "Green"=162, "Blue"=162}, {"Red"=163, "Green"=163, "Blue"=163}, {"Red"=164, "Green"=164, "Blue"=164}, {"Red"=165, "Green"=165, "Blue"=165}, {"Red"=166, "Green"=166, "Blue"=166}, {"Red"=167, "Green"=167, "Blue"=167}, {"Red"=168, "Green"=168, "Blue"=168}, {"Red"=169, "Green"=169, "Blue"=169}, {"Red"=170, "Green"=170, "Blue"=170}, {"Red"=171, "Green"=171, "Blue"=171}, {"Red"=172, "Green"=172, "Blue"=172}, {"Red"=173, "Green"=173, "Blue"=173}, {"Red"=174, "Green"=174, "Blue"=174}, {"Red"=175, "Green"=175, "Blue"=175}, {"Red"=176, "Green"=176, "Blue"=176}, {"Red"=177, "Green"=177, "Blue"=177}, {"Red"=178, "Green"=178, "Blue"=178}, {"Red"=179, "Green"=179, "Blue"=179}, {"Red"=180, "Green"=180, "Blue"=180}, {"Red"=181, "Green"=181, "Blue"=181}, {"Red"=182, "Green"=182, "Blue"=182}, {"Red"=183, "Green"=183, "Blue"=183}, {"Red"=184, "Green"=184, "Blue"=184}, {"Red"=185, "Green"=185, "Blue"=185}, {"Red"=186, "Green"=186, "Blue"=186}, {"Red"=187, "Green"=187, "Blue"=187}, {"Red"=188, "Green"=188, "Blue"=188}, {"Red"=189, "Green"=189, "Blue"=189}, {"Red"=190, "Green"=190, "Blue"=190}, {"Red"=191, "Green"=191, "Blue"=191}, {"Red"=192, "Green"=192, "Blue"=192}, {"Red"=193, "Green"=193, "Blue"=193}, {"Red"=194, "Green"=194, "Blue"=194}, {"Red"=195, "Green"=195, "Blue"=195}, {"Red"=196, "Green"=196, "Blue"=196}, {"Red"=197, "Green"=197, "Blue"=197}, {"Red"=198, "Green"=198, "Blue"=198}, {"Red"=199, "Green"=199, "Blue"=199}, {"Red"=200, "Green"=200, "Blue"=200}, {"Red"=201, "Green"=201, "Blue"=201}, {"Red"=202, "Green"=202, "Blue"=202}, {"Red"=203, "Green"=203, "Blue"=203}, {"Red"=204, "Green"=204, "Blue"=204}, {"Red"=205, "Green"=205, "Blue"=205}, {"Red"=206, "Green"=206, "Blue"=206}, {"Red"=207, "Green"=207, "Blue"=207}, {"Red"=208, "Green"=208, "Blue"=208}, {"Red"=209, "Green"=209, "Blue"=209}, {"Red"=210, "Green"=210, "Blue"=210}, {"Red"=211, "Green"=211, "Blue"=211}, {"Red"=212, "Green"=212, "Blue"=212}, {"Red"=213, "Green"=213, "Blue"=213}, {"Red"=214, "Green"=214, "Blue"=214}, {"Red"=215, "Green"=215, "Blue"=215}, {"Red"=216, "Green"=216, "Blue"=216}, {"Red"=217, "Green"=217, "Blue"=217}, {"Red"=218, "Green"=218, "Blue"=218}, {"Red"=219, "Green"=219, "Blue"=219}, {"Red"=220, "Green"=220, "Blue"=220}, {"Red"=221, "Green"=221, "Blue"=221}, {"Red"=222, "Green"=222, "Blue"=222}, {"Red"=223, "Green"=223, "Blue"=223}, {"Red"=224, "Green"=224, "Blue"=224}, {"Red"=225, "Green"=225, "Blue"=225}, {"Red"=226, "Green"=226, "Blue"=226}, {"Red"=227, "Green"=227, "Blue"=227}, {"Red"=228, "Green"=228, "Blue"=228}, {"Red"=229, "Green"=229, "Blue"=229}, {"Red"=230, "Green"=230, "Blue"=230}, {"Red"=231, "Green"=231, "Blue"=231}, {"Red"=232, "Green"=232, "Blue"=232}, {"Red"=233, "Green"=233, "Blue"=233}, {"Red"=234, "Green"=234, "Blue"=234}, {"Red"=235, "Green"=235, "Blue"=235}, {"Red"=236, "Green"=236, "Blue"=236}, {"Red"=237, "Green"=237, "Blue"=237}, {"Red"=238, "Green"=238, "Blue"=238}, {"Red"=239, "Green"=239, "Blue"=239}, {"Red"=240, "Green"=240, "Blue"=240}, {"Red"=241, "Green"=241, "Blue"=241}, {"Red"=242, "Green"=242, "Blue"=242}, {"Red"=243, "Green"=243, "Blue"=243}, {"Red"=244, "Green"=244, "Blue"=244}, {"Red"=245, "Green"=245, "Blue"=245}, {"Red"=246, "Green"=246, "Blue"=246}, {"Red"=247, "Green"=247, "Blue"=247}, {"Red"=248, "Green"=248, "Blue"=248}, {"Red"=249, "Green"=249, "Blue"=249}, {"Red"=250, "Green"=250, "Blue"=250}, {"Red"=251, "Green"=251, "Blue"=251}, {"Red"=252, "Green"=252, "Blue"=252}, {"Red"=253, "Green"=253, "Blue"=253}, {"Red"=254, "Green"=254, "Blue"=254}, {"Red"=255, "Green"=255, "Blue"=255}] ("Color Palette")] -> w101
              frame "high clipping red" {
              }
              frame "low clipping blue" {
              }
              frame "high and low clipping" {
              }
              frame "standard" {
              }
            }
            n67 = call-poly "GFGpolyGet.vi"() -> ("error out"=w109:errorcluster, "DisplayRefsOut(generic class)"=w108:T14)  [unwired: 10 in]
            n68 = Cluster To Array(cluster=w108) -> (array=w106:refnum<vi>[])
            n69 = for {
              tunnel: w106 -> [w116] mode=indexing
              tunnel: w101 -> [w120]
              tunnel: w105 -> [w119]
              tunnel: w109 -> [w118]
              tunnel: [w117] -> _
              tunnel: w107 -> [w114]
              n70 = To More Specific Class(target class=w114, reference=w116) -> (specific class reference=w115:refnum<vi>)  [unwired: 1 in, 1 out]
              n71 = property class="ImageControl"(reference=w115, error in=w118, "User Palette"=w120, "Palette Type"=w119) -> (error out=w117:errorcluster)  [unwired: 1 out]
            }
          }
          frame "display.queue.to.fp.display_MD.completed", "galvo.scan.engine_MD.completed", "image.queue.to.disk.and.display.queue_MD.completed", "raw.queue.to.image.queue_MD.completed" {
            n72 = for {
              N: 1 -> [_]
              shift-right: [w135] -> _
              shift-left: _ -> [w137]
              tunnel: [w136] -> w128
              n73 = Tick Count (ms)() -> (millisecond timer value=w135:u32)
              n74 = Subtract(x=w135, y=w137) -> (x-y=w136:u32)
            }
            n75 = Greater?(x=u32 500 ("y"), y=w128) -> (0:w125:bool)
            n76 = local read "String"() -> (w124:string)
            n77 = Select(t=w124, s=w125, f="") -> (s? t:f=w126:string)
            n78 = Concatenate Strings(w126, "\r\n", w122) -> (w133:string)
            n79 = for {
              tunnel: w133 -> [w144]
              tunnel: string[] ["galvo.scan.engine_MD.completed", "raw.queue.to.image.queue_MD.completed", "image.queue.to.disk.and.display.queue_MD.completed", "display.queue.to.fp.display_MD.completed"] ("appended array") -> [w143] mode=indexing
              shift-right: [w139] -> w130
              shift-left: i16 0 -> [w138]
              n80 = Match Pattern(string=w144, regular expression=w143) -> (offset past match=w142:i32)  [unwired: 1 in, 3 out]
              n81 = Greater Or Equal To 0?(x=w142) -> (x >= 0?=w141:bool)
              n82 = Boolean To (0,1)(Boolean=w141) -> (0, 1=w140:i16)
              n83 = Add(x=w140, y=w138) -> (x+y=w139:i16)
            }
            n84 = local write "String"(w133) -> ()
            n85 = disable-structure shown="Enabled" {
              disable-tunnel: w130 -> [w146 _]
              frame Enabled {
                n86 = Equal?(x=w146, y=4) -> (x = y?=w145:bool)
                n87 = case shown="True" w145 {
                  selector: w145 -> [_ w148]
                  frame False {
                  }
                  frame True {
                    n88 = call "GFG_core.vi"("Variable Name in"="flystop", "Variant in"=FALSE ("x = y?"), "Action"=enum16{"Init", "Set", "Get"}."Set") -> ()  [unwired: 10 in, 7 out]
                    n89 = local write "String"("") -> ()
                    "ready for flystart?" <- w148
                  }
                }
              }
              frame Disabled {
              }
            }
          }
          frame "ROTATE", "Start.Delay", "fill.fraction", "max.field.of.view", "nomin.x.pixels", "pixel.dwell.time.in.sec", "rotate.enable", "voltage.for.max.field.of.view", "x.bidirectional", "x.volt.offset", "y.bidirectional", "y.pixels", "y.volt.offset" {
            n90 = for {
              N: 1 -> [_]
              tunnel: [w166] -> w155 mode=indexing
              shift-right: [w162] -> _
              shift-left: _ -> [w164]
              tunnel: [w161] -> w153
              n91 = Tick Count (ms)() -> (millisecond timer value=w162:u32)
              n92 = Subtract(x=w162, y=w164) -> (x-y=w165:u32)
              n93 = Greater?(x=w165, y=u32 500) -> (0:w161:bool)
              n94 = case shown="True" w161 {
                tunnel: [_ w169] -> w166
                frame False {
                }
                frame True {
                  n95 = call-poly "GFGpolyGet.vi"("Variable Name in"="FOCUS") -> ("Boolean"=w167:bool)  [unwired: 10 in]
                  n96 = case shown="True" w167 {
                    frame False {
                    }
                    frame True {
                      n97 = call "kill task and queues for flystart.vi"() -> ()  [unwired: 12 in]
                    }
                  }
                  n98 = call "GFG_core.vi"("Variable Name in"="flystop", "Variant in"=w167, "Action"=enum16{"Init", "Set", "Get"}."Set") -> ("error out"=w169:errorcluster)  [unwired: 10 in, 6 out]
                  n99 = Wait (ms)(milliseconds to wait=u32 50) -> ()  [unwired: 1 out]
                }
              }
            }
            n100 = case shown="\"False\", Default" w160 {
              tunnel: w159 -> [_ w211 _ _]
              tunnel: w158 -> [_ _ w234 _]
              tunnel: w157 -> [_ _ _ w241]
              tunnel: w155 -> [_ _ _ _]
              tunnel: w153 -> [w173 _ _ _]
              frame "False", Default {
                n101 = case shown="True" w173 {
                  frame False {
                  }
                  frame True {
                    n102 = call-poly "GFGpolyGet.vi"("Variable Name in"="y.pixels") -> ("Numeric"=w178:dbl)  [unwired: 9 in, 1 out]
                    n103 = call-poly "GFGpolyGet.vi"("Variable Name in"="max.field.of.view") -> ("Numeric"=w193:dbl)  [unwired: 9 in, 1 out]
                    n104 = call-poly "GFGpolyGet.vi"("Variable Name in"="ZOOM") -> ("Numeric"=w192:dbl)  [unwired: 9 in, 1 out]
                    n105 = Divide(x=w193, y=w192) -> (x/y=w184:dbl)
                    n106 = call-poly "GFGpolyGet.vi"("Variable Name in"="nomin.x.pixels") -> ("Numeric"=w180:dbl)  [unwired: 9 in, 1 out]
                    n107 = call "GFG_core.vi"("Variable Name in"="pixel.resolution") -> ("Variant Out"=w175:variant)  [unwired: 12 in, 6 out]
                    n108 = call-poly "GFGpolyGet.vi"("Variable Name in"="fill.fraction") -> ("Numeric"=w190:dbl)  [unwired: 9 in, 1 out]
                    n109 = Build Array(w180, w178) -> (w183:dbl[])
                    n110 = Variant To Data(type=pixel_resolution_enum."   128 x 128" ("pixel resolution"), Variant=w175) -> (data=w174:T3)  [unwired: 1 in, 1 out]
                    n111 = Divide(x=w190, y=100.0) -> (x/y=w188:dbl)
                    n112 = Divide(x=w180, y=w188) -> (x/y=w185:dbl)
                    n113 = Array Max & Min(array=w183) -> (max value=w182:dbl)  [unwired: 3 out]
                    n114 = call "GFG_core.vi"("Variable Name in"="x.pixels", "Variant in"=w185, "Action"=enum16{"Init", "Set", "Get"}."Set") -> ()  [unwired: 10 in, 7 out]
                    n115 = case shown="\"   arbitrary\"" w174 {
                      tunnel: w184 -> [_ w198]
                      tunnel: w182 -> [_ w196]
                      frame "   arbitrary" {
                      }
                      frame "   256 x 128", Default {
                        n116 = Divide(x=w198, y=w196) -> (x/y=w197:dbl)
                        n117 = call "GFG_core.vi"("Variable Name in"="x.pixel.sz", "Variant in"=w197, "Action"=enum16{"Init", "Set", "Get"}."Set") -> ()  [unwired: 10 in, 7 out]
                        n118 = call "GFG_core.vi"("Variable Name in"="y.pixel.sz", "Variant in"=w197, "Action"=enum16{"Init", "Set", "Get"}."Set") -> ()  [unwired: 10 in, 7 out]
                      }
                    }
                  }
                }
              }
              frame "x.bidirectional" {
                n119 = Variant To Data(type=TRUE, Variant=w211) -> (data=w204:bool)  [unwired: 1 in, 1 out]
                n120 = call-poly "GFGpolyGet.vi"("Variable Name in"="speed mode") -> ("output cluster"=w208:T13)  [unwired: 9 in, 1 out]
                n121 = call "GFG_core.vi"("Variable Name in"="scan mode main settings") -> ("Variant Out"=w214:variant)  [unwired: 12 in, 6 out]
                n122 = Unbundle By Name(w208) -> ("RingRef"=w207:refnum<vi>)
                n123 = Variant To Data(type=scan_mode_main_settings_tab."2D line scan" ("scan mode main settings"), Variant=w214) -> (data=w212:T1)  [unwired: 1 in, 1 out]
                n124 = case shown="\"2D frame\", Default" w212 {
                  tunnel: w204 -> [w221 _]
                  frame "2D frame", Default {
                    n125 = call-poly "GFGpolyGet.vi"("Variable Name in"="MAIN Image panels ") -> ("output cluster"=w217:T13)  [unwired: 9 in, 1 out]
                    n126 = call "GFG_core.vi"("Variable Name in"="fill.fraction.bidi") -> ("Variant Out"=w223:variant)  [unwired: 12 in, 6 out]
                    n127 = Unbundle By Name(w217) -> ("TabControlRef"=w219:refnum<vi>)
                    n128 = call "GFG_core.vi"("Variable Name in"="fill.fraction.unidi") -> ("Variant Out"=w224:variant)  [unwired: 12 in, 6 out]
                    n129 = Select(t=w223, s=w221, f=w224) -> (s? t:f=w222:variant)
                    n130 = call "GFG_core.vi"("Variable Name in"="fill.fraction", "Variant in"=w222, "Action"=enum16{"Init", "Set", "Get"}."Set") -> ()  [unwired: 10 in, 7 out]
                    n131 = property class="TabCtl"(reference=w219, "Tabs Visible?"=TRUE) -> ()  [unwired: 1 in, 2 out]
                    n132 = call "GFG refresh all variables.vi"("All Variable Names"=string[] ["pixel resolution"]) -> ()  [unwired: 11 in]
                  }
                  frame "2D line scan" {
                    n133 = call "GFG_core.vi"("Variable Name in"="fill.fraction.line", "Action"=enum16{"Init", "Set", "Get"}."Get") -> ("Variant Out"=w229:variant)  [unwired: 11 in, 6 out]
                    n134 = call "GFG_core.vi"("Variable Name in"="fill.fraction", "Variant in"=w229, "Action"=enum16{"Init", "Set", "Get"}."Set") -> ()  [unwired: 10 in, 7 out]
                  }
                }
                n135 = Select(t=i32[] [] ("Disabled Items []"), s=w204, f=i32[] [0, 1] ("Disabled Items []")) -> (s? t:f=w203:i32[])
                n136 = property class="Ring"(reference=w207, "Disabled Items []"=w203) -> ()  [unwired: 1 in, 2 out]
              }
              frame "pixel.dwell.time.in.sec." {
                n137 = call "GFG_core.vi"("Variable Name in"="scan mode main settings") -> ("Variant Out"=w237:variant)  [unwired: 12 in, 6 out]
                n138 = Variant To Data(type=scan_mode_main_settings_tab."2D line scan" ("scan mode main settings"), Variant=w237) -> (data=w235:T1)  [unwired: 1 in, 1 out]
                n139 = case shown="\"2D frame\", Default" w235 {
                  tunnel: [5 w240] -> _
                  tunnel: w234 -> [_ w240]
                  frame "2D frame", Default {
                  }
                  frame "2D line scan" {
                  }
                }
              }
              frame "fill.fraction" {
                n140 = call "getVIname.vi"() -> ("VI name"=w242:string)  [unwired: 19 in]
                n141 = Not Equal?(x=w242, y=w241) -> (x != y?=w243:bool)
                n142 = case shown="True" w243 {
                  frame False {
                  }
                  frame True {
                    n143 = call "GFG_core.vi"("Variable Name in"="x.bidirectional") -> ("Variant Out"=w250:variant)  [unwired: 12 in, 6 out]
                    n144 = call "GFG_core.vi"("Variable Name in"="scan mode main settings") -> ("Variant Out"=w247:variant)  [unwired: 12 in, 6 out]
                    n145 = Variant To Data(type=TRUE, Variant=w250) -> (data=w249:bool)  [unwired: 1 in, 1 out]
                    n146 = Variant To Data(type=scan_mode_main_settings_tab."2D line scan" ("scan mode main settings"), Variant=w247) -> (data=w244:T1)  [unwired: 1 in, 1 out]
                    n147 = case shown="\"2D frame\", Default" w244 {
                      tunnel: w249 -> [w252 _]
                      frame "2D frame", Default {
                        n148 = case shown="False" w252 {
                          frame False {
                            n149 = call "GFG_core.vi"("Variable Name in"="fill.fraction") -> ("Variant Out"=w253:variant)  [unwired: 12 in, 6 out]
                            n150 = call "GFG_core.vi"("Variable Name in"="fill.fraction.unidi", "Variant in"=w253, "Action"=enum16{"Init", "Set", "Get"}."Set") -> ()  [unwired: 10 in, 7 out]
                          }
                          frame True {
                            n151 = call "GFG_core.vi"("Variable Name in"="fill.fraction") -> ("Variant Out"=w257:variant)  [unwired: 12 in, 6 out]
                            n152 = call "GFG_core.vi"("Variable Name in"="fill.fraction.bidi", "Variant in"=w257, "Action"=enum16{"Init", "Set", "Get"}."Set") -> ()  [unwired: 10 in, 7 out]
                          }
                        }
                      }
                      frame "2D line scan" {
                      }
                    }
                  }
                }
              }
            }
          }
          frame "x.pixel.sz", "y.pixel.sz" {
          }
          frame "no..of.frames.to.acquire" {
            n153 = Variant To Data(type=0.0, Variant=w269) -> (data=w263:dbl)  [unwired: 1 in, 1 out]
            n154 = call-poly "GFGpolyGet.vi"("Variable Name in"="frame count") -> ("output cluster"=w271:T13)  [unwired: 9 in, 1 out]
            n155 = call "GFG_core.vi"("Variable Name in"="scan mode main settings") -> ("Variant Out"=w265:variant)  [unwired: 12 in, 6 out]
            n156 = Unbundle By Name(w271) -> ("SlideRef"=w270:refnum<vi>)
            n157 = Variant To Data(type=scan_mode_main_settings_tab."2D line scan" ("scan mode main settings"), Variant=w265) -> (data=w262:T1)  [unwired: 1 in, 1 out]
            n158 = property class="Slide"(reference=w270, "Scale.Maximum"=w263) -> ()  [unwired: 1 in, 2 out]
            n159 = case shown="\"2D frame\", Default" w262 {
              tunnel: w263 -> [w273 _]
              frame "2D frame", Default {
                n160 = call "GFG_core.vi"("Variable Name in"="no.of.frames.for.frame.scan", "Variant in"=w273, "Action"=enum16{"Init", "Set", "Get"}."Set") -> ()  [unwired: 10 in, 7 out]
              }
              frame "2D line scan" {
              }
            }
          }
          frame "reset.zoom" {
            n161 = call-poly "GFGpolyGet.vi"() -> ("DisplayRefsOut(generic class)"=w281:T14)  [unwired: 10 in, 1 out]
            n162 = call-poly "GFGpolyGet.vi"() -> ("Image Refs Out"=w280:T16)  [unwired: 10 in, 1 out]
            n163 = Cluster To Array(cluster=w281) -> (array=w279:refnum<vi>[])
            n164 = Cluster To Array(cluster=w280) -> (array=w278:T15[])
            n165 = call "set initial zoom.vi"("reset?"=TRUE, "Image Refs In"=w278, "DisplayRefsIn(generic class)"=w279) -> ()  [unwired: 9 in]
          }
          frame "ZOOM", "pixel.resolution", "speed.mode" {
            n166 = for {
              N: 1 -> [_]
              tunnel: [w293] -> w282 mode=indexing
              shift-right: [w288] -> _
              shift-left: _ -> [w291]
              n167 = Tick Count (ms)() -> (millisecond timer value=w288:u32)
              n168 = Subtract(x=w288, y=w291) -> (x-y=w292:u32)
              n169 = Greater?(x=w292, y=u32 500) -> (0:w289:bool)
              n170 = case shown="True" w289 {
                tunnel: [_ w296] -> w293
                frame False {
                }
                frame True {
                  n171 = call-poly "GFGpolyGet.vi"("Variable Name in"="FOCUS") -> ("Boolean"=w294:bool)  [unwired: 10 in]
                  n172 = case shown="True" w294 {
                    frame False {
                    }
                    frame True {
                      n173 = call "kill task and queues for flystart.vi"() -> ()  [unwired: 12 in]
                    }
                  }
                  n174 = call "GFG_core.vi"("Variable Name in"="flystop", "Variant in"=w294, "Action"=enum16{"Init", "Set", "Get"}."Set") -> ("error out"=w296:errorcluster)  [unwired: 10 in, 6 out]
                  n175 = Wait (ms)(milliseconds to wait=u32 50) -> ()  [unwired: 1 out]
                }
              }
            }
            n176 = case shown="\"pixel.resolution\"" w285 {
              tunnel: w287 -> [_ w306]
              tunnel: [w300 w304] -> w286
              tunnel: w282 -> [_ _]
              frame "ZOOM", Default {
                n177 = call "GFG_core.vi"("Variable Name in"="pixel.resolution") -> ("Variant Out"=w302:variant)  [unwired: 12 in, 6 out]
                n178 = Variant To Data(type=pixel_resolution_enum."   128 x 128" ("pixel resolution"), Variant=w302) -> (data=w300:T3)  [unwired: 1 in, 1 out]
              }
              frame "pixel.resolution" {
                n179 = Variant To Data(type=pixel_resolution_enum."   128 x 128" ("pixel resolution"), Variant=w306) -> (data=w304:T3)  [unwired: 1 in, 1 out]
              }
            }
            n180 = case shown="\"   arbitrary\"" w286 {
              selector: w286 -> [_ w330]
              frame "   arbitrary" {
                w310 = "nomin.x.pixels" ("Variable Name in")
                n181 = call-poly "GFGpolyGet.vi"("Variable Name in"="ZOOM") -> ("output cluster"=w315:T13)  [unwired: 9 in, 1 out]
                n182 = call-poly "GFGpolyGet.vi"("Variable Name in"="speed.mode") -> ("output cluster"=w320:T13)  [unwired: 9 in, 1 out]
                n183 = Build Array("nomin.x.pixels" ("Variable Name in"), "y.pixel.sz" ("Variable Name in"), "x.pixel.sz" ("Variable Name in"), "pixel.dwell.time.in.sec" ("Variable Name in"), "y.pixels" ("Variable Name in")) -> (w321:string[])
                n184 = Unbundle By Name(w315) -> ("SlideRef"=w317:refnum<vi>)
                n185 = Unbundle By Name(w320) -> ("RingRef"=w318:refnum<vi>)
                n186 = property class="Slide"(reference=w317, "DisabledEnum"=T4."Disabled and Grayed Out" ("Disabled")) -> ()  [unwired: 1 in, 2 out]
                n187 = for {
                  tunnel: w321 -> [w328] mode=indexing
                  n188 = call-poly "GFGpolyGet.vi"("Variable Name in"=w328) -> ("output cluster"=w327:T13)  [unwired: 9 in, 1 out]
                  n189 = Unbundle By Name(w327) -> ("DigitalRef"=w325:refnum<vi>)
                  n190 = property class="DigNum"(reference=w325, "DisabledEnum"=T4."Enabled" ("Disabled")) -> ()  [unwired: 1 in, 2 out]
                }
                n191 = property class="Ring"(reference=w318, "DisabledEnum"=T4."Disabled and Grayed Out" ("Disabled")) -> ()  [unwired: 1 in, 2 out]
                n192 = call "GFG_core.vi"("Variable Name in"=w310, "Action"=enum16{"Init", "Set", "Get"}."Get") -> ("Variant Out"=w309:variant)  [unwired: 11 in, 6 out]
                n193 = call "GFG_core.vi"("Variable Name in"=w310, "Variant in"=w309, "Action"=enum16{"Init", "Set", "Get"}."Set") -> ()  [unwired: 10 in, 7 out]
              }
              frame Default {
                w359 = T17 0 items=["high-speed scan", "standard scan", "long exposure"] ("speed mode")
                n194 = Build Array("nomin.x.pixels" ("Variable Name in"), "y.pixel.sz" ("Variable Name in"), "x.pixel.sz" ("Variable Name in"), "pixel.dwell.time.in.sec" ("Variable Name in"), "y.pixels" ("Variable Name in")) -> (w369:string[])
                n195 = call "GFG_core.vi"("Variable Name in"="speed.mode") -> ("Variant Out"=w358:variant)  [unwired: 12 in, 6 out]
                n196 = for {
                  tunnel: w369 -> [w403] mode=indexing
                  n197 = call-poly "GFGpolyGet.vi"("Variable Name in"=w403) -> ("output cluster"=w402:T13)  [unwired: 9 in, 1 out]
                  n198 = Unbundle By Name(w402) -> ("DigitalRef"=w400:refnum<vi>)
                  n199 = property class="DigNum"(reference=w400, "DisabledEnum"=T4."Disabled and Grayed Out" ("Disabled")) -> (error out=→"error out 2":errorcluster)  [unwired: 1 in, 1 out]
                }
                n200 = Variant To Data(type=w359, Variant=w358) -> (data=w334:T17)  [unwired: 1 in, 1 out]
                n201 = case shown="\"   512 x  64\"" w330 {
                  tunnel: [128 256 256 512 512 512 512 1024 1024] -> w332
                  tunnel: [128 128 256 256 128 64 512 512 1024] -> w331
                  frame "   128 x 128", Default {
                  }
                  frame "   256 x 128" {
                  }
                  frame "   256 x 256" {
                  }
                  frame "   512 x 256" {
                  }
                  frame "   512 x 128" {
                  }
                  frame "   512 x  64" {
                  }
                  frame "   512 x 512" {
                  }
                  frame "  1024 x 512" {
                  }
                  frame "  1024 x 1024" {
                  }
                }
                n202 = case shown="0, Default" w334 {
                  tunnel: [1e-06 2e-06 4e-06 8e-06] -> w335
                  frame 0, Default {
                  }
                  frame 1 {
                  }
                  frame 2 {
                  }
                  frame 3 {
                  }
                }
                n203 = call "GFG_core.vi"("Variable Name in"="pixel.dwell.time.in.sec", "Variant in"=w335, "Action"=enum16{"Init", "Set", "Get"}."Set") -> ()  [unwired: 10 in, 7 out]
                n204 = call-poly "GFGpolyGet.vi"("Variable Name in"="max.field.of.view") -> ("Numeric"=w354:dbl)  [unwired: 9 in, 1 out]
                n205 = call "GFG_core.vi"("Variable Name in"="y.pixels", "Variant in"=w331, "Action"=enum16{"Init", "Set", "Get"}."Set") -> ()  [unwired: 10 in, 7 out]
                n206 = call-poly "GFGpolyGet.vi"("Variable Name in"="ZOOM") -> ("Numeric"=w353:dbl)  [unwired: 9 in, 1 out]
                n207 = call "GFG_core.vi"("Variable Name in"="nomin.x.pixels", "Variant in"=w332, "Action"=enum16{"Init", "Set", "Get"}."Set") -> ()  [unwired: 10 in, 7 out]
                n208 = Divide(x=w354, y=w353) -> (x/y=w341:dbl)
                n209 = call-poly "GFGpolyGet.vi"("Variable Name in"="fill.fraction") -> ("Numeric"=w347:dbl)  [unwired: 9 in, 1 out]
                n210 = Build Array(w332, w331) -> (w339:i32[])
                n211 = Divide(x=w347, y=100.0) -> (x/y=w345:dbl)
                n212 = call-poly "GFGpolyGet.vi"("Variable Name in"="ZOOM") -> ("output cluster"=w362:T13)  [unwired: 9 in, 1 out]
                n213 = call-poly "GFGpolyGet.vi"("Variable Name in"="speed.mode") -> ("output cluster"=w367:T13)  [unwired: 9 in, 1 out]
                n214 = Divide(x=w332, y=w345) -> (x/y=w342:dbl)
                n215 = Unbundle By Name(w362) -> ("SlideRef"=w364:refnum<vi>)
                n216 = Unbundle By Name(w367) -> ("RingRef"=w365:refnum<vi>)
                n217 = Array Max & Min(array=w339) -> (max value=w338:i32)  [unwired: 3 out]
                n218 = call "GFG_core.vi"("Variable Name in"="x.pixels", "Variant in"=w342, "Action"=enum16{"Init", "Set", "Get"}."Set") -> ()  [unwired: 10 in, 7 out]
                n219 = property class="Slide"(reference=w364, "DisabledEnum"=T4."Enabled" ("Disabled")) -> ()  [unwired: 1 in, 2 out]
                n220 = Divide(x=w341, y=w338) -> (x/y=w340:dbl)
                n221 = property class="Ring"(reference=w365, "DisabledEnum"=T4."Enabled" ("Disabled")) -> (error out=→"error out":errorcluster)  [unwired: 1 in, 1 out]
                n222 = call "GFG_core.vi"("Variable Name in"="x.pixel.sz", "Variant in"=w340, "Action"=enum16{"Init", "Set", "Get"}."Set") -> ()  [unwired: 10 in, 7 out]
                n223 = call "GFG_core.vi"("Variable Name in"="y.pixel.sz", "Variant in"=w340, "Action"=enum16{"Init", "Set", "Get"}."Set") -> ()  [unwired: 10 in, 7 out]
              }
            }
          }
          frame "piezo.mode" {
            n224 = call-poly "GFGpolyGet.vi"("Variable Name in"="frames.per.z.cycle") -> ("output cluster"=w412:T13)  [unwired: 9 in, 1 out]
            n225 = call-poly "GFGpolyGet.vi"("Variable Name in"="piezo.mode") -> ("Boolean"=w406:bool)  [unwired: 10 in]
            n226 = Unbundle By Name(w412) -> ("DigitalRef"=w411:refnum<vi>)
            n227 = Select(t=T6 {"Minimum"=3.0, "Maximum"=101.0, "Increment"=2.0} ("Data Entry Limits"), s=w406, f=T6 {"Minimum"=4.0, "Maximum"=100.0, "Increment"=2.0} ("Data Entry Limits")) -> (s? t:f=w407:T6)
            n228 = property class="DigNum"(reference=w411, "Data Range"=w407, "OutOfRngAction"=T5 {"Out of Range Action Minimum"=1, "Out of Range Action Maximum"=1, "Out of Range Action Increment"=1} ("Response to Value Outside Limits")) -> ()  [unwired: 1 in, 2 out]
          }
          frame "scan.mode.main.settings" {
            n229 = Variant To Data(type=scan_mode_main_settings_tab."2D frame" ("scan mode main settings"), Variant=w418) -> (data=w416:T1)  [unwired: 1 in, 1 out]
            n230 = case shown="\"2D frame\", Default" w416 {
              tunnel: w415 -> [w455 w462 w469]
              tunnel: [w455 w462 w469] -> w414
              frame "2D frame", Default {
                w419 = enum16{"Init", "Set", "Get"}."Set" ("Action")
                n231 = call-poly "GFGpolyGet.vi"("Variable Name in"="y.pixels") -> ("output cluster"=w446:T13)  [unwired: 9 in, 1 out]
                n232 = Unbundle By Name(w446) -> ("DigitalRef"=w445:refnum<vi>)
                n233 = call "GFG refresh all variables.vi"("All Variable Names"=string[] ["pixel resolution", "x.bidirectional"]) -> ()  [unwired: 11 in]
                n234 = property class="DigNum"(reference=w445, "DisabledEnum"=T4."Enabled" ("Disabled")) -> ()  [unwired: 1 in, 2 out]
                n235 = call-poly "GFGpolyGet.vi"("Variable Name in"="fill.fraction") -> ("output cluster"=w443:T13)  [unwired: 9 in, 1 out]
                n236 = call "GFG_core.vi"("Variable Name in"="no..of.frames.for.frame.scan", "Action"=enum16{"Init", "Set", "Get"}."Get") -> ("Variable Name Out"=w449:string)  [unwired: 11 in, 6 out]
                n237 = Unbundle By Name(w443) -> ("DigitalRef"=w444:refnum<vi>)
                n238 = call "GFG_core.vi"("Variable Name in"=" no..of.frames.to.acquire", "Variant in"=w449, "Action"=enum16{"Init", "Set", "Get"}."Set") -> ()  [unwired: 10 in, 7 out]
                n239 = property class="DigNum"(reference=w444, "DisabledEnum"=T4."Enabled" ("Disabled")) -> ()  [unwired: 1 in, 2 out]
                n240 = call "GFG_core.vi"("Variable Name in"="experiment type", "Variant in"=T8 "XYT" ("experiment type"), "Action"=enum16{"Init", "Set", "Get"}."Set") -> ()  [unwired: 10 in, 7 out]
                n241 = call "GFG_core.vi"("Variable Name in"="xy.voltage.map") -> ("Variant Out"=w435:variant)  [unwired: 12 in, 6 out]
                n242 = call "line scan enable disable.vi"("Page Enabled State"=T9."Page Disabled & Grayed") -> ()  [unwired: 11 in]
                n243 = Variant To Data(type=T7 {"xyvoltagefor2frames"=[], "x.pixels"=0.0, "nomin.x.pixels"=0.0, "y.pixels"=0.0, "fill.fraction"=0.0, "x.bidirectional"=FALSE, "y.bidirectional"=FALSE} ("output cluster"), Variant=w435) -> (data=w432:T7, error out=→"error out 3":errorcluster)  [unwired: 1 in]
                n244 = Unbundle(w432) -> ("x.pixels"=w430:dbl, "nomin.x.pixels"=w428:dbl, "y.pixels"=w426:dbl, "fill.fraction"=w424:dbl, "x.bidirectional"=w422:bool, "y.bidirectional"=w420:bool)  [unwired: 1 out]
                n245 = call "GFG_core.vi"("Variable Name in"="x.pixels" ("Tag in"), "Variant in"=w430, "Action"=w419) -> ()  [unwired: 10 in, 7 out]
                n246 = call "GFG_core.vi"("Variable Name in"="nomin.x.pixels", "Variant in"=w428, "Action"=w419) -> ()  [unwired: 10 in, 7 out]
                n247 = call "GFG_core.vi"("Variable Name in"="y.pixels" ("Tag in"), "Variant in"=w426, "Action"=w419) -> ()  [unwired: 10 in, 7 out]
                n248 = call "GFG_core.vi"("Variable Name in"="fill.fraction", "Variant in"=w424, "Action"=w419) -> ()  [unwired: 10 in, 7 out]
                n249 = call "GFG_core.vi"("Variable Name in"="x.bidirectional" ("Tag in"), "Variant in"=w422, "Action"=w419) -> ()  [unwired: 10 in, 7 out]
                n250 = call "GFG_core.vi"("Variable Name in"="y.bidirectional" ("Tag in"), "Variant in"=w420, "Action"=w419) -> ()  [unwired: 10 in, 7 out]
              }
              frame "Z Stack" {
                n251 = call "GFG_core.vi"("Variable Name in"="advanced settings inner tab", "Variant in"=advanced_settings_inner_tab_CTL."Zstack data" ("advanced settings inner tab"), "Action"=enum16{"Init", "Set", "Get"}."Set") -> ()  [unwired: 10 in, 7 out]
                n252 = call "GFG_core.vi"("Variable Name in"="experiment type", "Variant in"=T8 "XYTZ" ("experiment type"), "Action"=enum16{"Init", "Set", "Get"}."Set") -> ()  [unwired: 10 in, 7 out]
                n253 = call "control tab sliding.vi"("close(T)/open(F)"=FALSE, "String"="advanced settings slider tab") -> ()  [unwired: 10 in]
                n254 = call "GFG refresh all variables.vi"("All Variable Names"=string[] ["frames.per.plane"]) -> ()  [unwired: 11 in]
              }
              frame "2D line scan" {
                n255 = call "GFG_core.vi"("Variable Name in"="experiment type", "Variant in"=T8 "[xy]T" ("experiment type"), "Action"=enum16{"Init", "Set", "Get"}."Set") -> ()  [unwired: 10 in, 7 out]
              }
            }
          }
          frame "MAIN.Image.panels." {
            n256 = Variant To Data(type=MAIN_Image_panel_tab_Control_type_def."Channel 1" ("MAIN Image panels"), Variant=w478) -> (data=w477:T11)  [unwired: 1 in, 1 out]
            n257 = case shown="\"Channel 1\", Default" w477 {
              tunnel: w476 -> [w480 w482 w484 w486 w492]
              tunnel: [w480 w482 w484 w486 w492] -> w475
              tunnel: [Histogram_tab."hist Ch 1" ("Histograms tab") Histogram_tab."hist Ch 2" ("Histograms tab") Histogram_tab."hist Ch 3" ("Histograms tab") Histogram_tab."hist Ch 4" ("Histograms tab") Histogram_tab."hist Ch 1" ("Histograms tab")] -> w470
              frame "Channel 1", Default {
              }
              frame "Channel 2" {
              }
              frame "Channel 3" {
              }
              frame "Channel 4" {
              }
              frame "all channels" {
                n258 = call-poly "GFGpolyGet.vi"() -> ("DisplayRefsOut(generic class)"=w491:T14)  [unwired: 10 in, 1 out]
                n259 = call-poly "GFGpolyGet.vi"() -> ("Image Refs Out"=w490:T16)  [unwired: 10 in, 1 out]
                n260 = Cluster To Array(cluster=w491) -> (array=w489:refnum<vi>[])
                n261 = Cluster To Array(cluster=w490) -> (array=w488:T15[])
                n262 = call "set initial zoom.vi"("reset?"=TRUE, "Image Refs In"=w488, "DisplayRefsIn(generic class)"=w489) -> ()  [unwired: 9 in]
              }
            }
            n263 = call-poly "GFGpolyGet.vi"("Variable Name in"="Histograms tab") -> ("output cluster"=w473:T13)  [unwired: 9 in, 1 out]
            n264 = Unbundle By Name(w473) -> ("TabControlRef"=w471:refnum<vi>)
            n265 = property class="TabCtl"(reference=w471, "Value"=w470) -> ()  [unwired: 1 in, 2 out]
          }
          frame "Objective" {
            n266 = Variant To Data(type=u16 0, Variant=w512) -> (data=w494:u16)  [unwired: 1 in, 1 out]
            n267 = Increment(x=w494) -> (x+1=w506:u16)
            n268 = Number To Decimal String(number=w506) -> (decimal integer string=w499:string)  [unwired: 1 in]
            n269 = call "GFG_core.vi"("Variable Name in"="active.objective", "Variant in"=w494, "Action"=enum16{"Init", "Set", "Get"}."Set") -> ()  [unwired: 10 in, 7 out]
            n270 = Concatenate Strings("obj", w499, ".max.field.of.view") -> (w507:string)
            n271 = Concatenate Strings("obj", w499, ".voltage.for.max.field.of.view") -> (w500:string)
            n272 = call-poly "GFGpolyGet.vi"("Variable Name in"=w507) -> ("Numeric"=w504:dbl)  [unwired: 9 in, 1 out]
            n273 = call-poly "GFGpolyGet.vi"("Variable Name in"=w500) -> ("Numeric"=w497:dbl)  [unwired: 9 in, 1 out]
            n274 = call "GFG_core.vi"("Variable Name in"="max.field.of.view", "Variant in"=w504, "Action"=enum16{"Init", "Set", "Get"}."Set") -> ()  [unwired: 10 in, 7 out]
            n275 = call "GFG_core.vi"("Variable Name in"="voltage.for.max.field.of.view", "Variant in"=w497, "Action"=enum16{"Init", "Set", "Get"}."Set") -> ()  [unwired: 10 in, 7 out]
          }
          frame "shutdown" {
          }
        }
      }
    }
  }
